vi "IHS.vi"() -> ()   [LabVIEW 2024]
doc: "This Labview program is made to run and administere the insect sampling system, using a Universal Robots UR-5 cobot. An Arduino Nano and the developd SRS system."
uses:
  SRS/controls/IHS_JKI.ctl
  <vilib>/userDefined/High Color/IMAQdx.ctl
  <vilib>/vision/Image Controls.llb/IMAQ Image.ctl
  <vilib>/addons/_JKI Toolkits/State Machine/_JKI_lib_State_Machine.llb/Select State(s)_err__jki_lib_state_machine.vi
  <vilib>/addons/_JKI Toolkits/State Machine/_JKI_lib_State_Machine.llb/Select State(s)_bool__jki_lib_state_machine.vi
  c074a71b-bfa2-4d9f-837e-66d7d0769231.vi
  <vilib>/addons/_JKI Toolkits/State Machine/_JKI_lib_State_Machine.llb/Periodic Trigger__ogtk__JKI-SM__jki_lib_state_machine.vi
  <vilib>/Utility/xml.llb/Write to XML File(string).vi
  <vilib>/vision/driver/NI_Vision_Acquisition_Software.lvlib
  <vilib>/vision/NI_Vision_Development_Module.lvlib
panel:
  in  "Force picture":bool
  in  "Force botton":bool
  in  "Simulate robot connection":bool
  in  "Training Picture":bool
  out "Num Before Next Pic":i32
  out "Executing Assignment":string
  out "Sample Num":i32
  in  "Save Settings":bool
  in  "Settings Button":bool
  out "Remote port":u16=30002
  out "UR-IP-address":string="192.168.0.10"
  out "Length":dbl
  out "CoM Y":dbl
  out "CoM X":dbl
  out "Orientation":dbl
  out "UR-Ready":bool
  out "Cam Connection":bool
  out "UR Connection":bool
  in  "Sample ID":string="Default"
  out "Robotmessage":string
  out "Number of objects":i32
  in  "Save Pictures":bool
  out "Vision A. Image":T1(plugin-control)
  out "Camera feed":T1(plugin-control)
  in  "Save Status His":bool
  out "Status History":string
  out "Insect-data-array":string[][](array[string])
  out "Status":string
  in  "Exit":bool
  in  "Pause Program":bool
  in  "Start Robot":bool
  # "Settings"
  # "Specimen info"
  # "-100°<RZ<100°"
  # "1.0mm<L<25.0mm"
  # "-0.750m<Y<0.750m"
  # "-0.750m<X<0.750m"
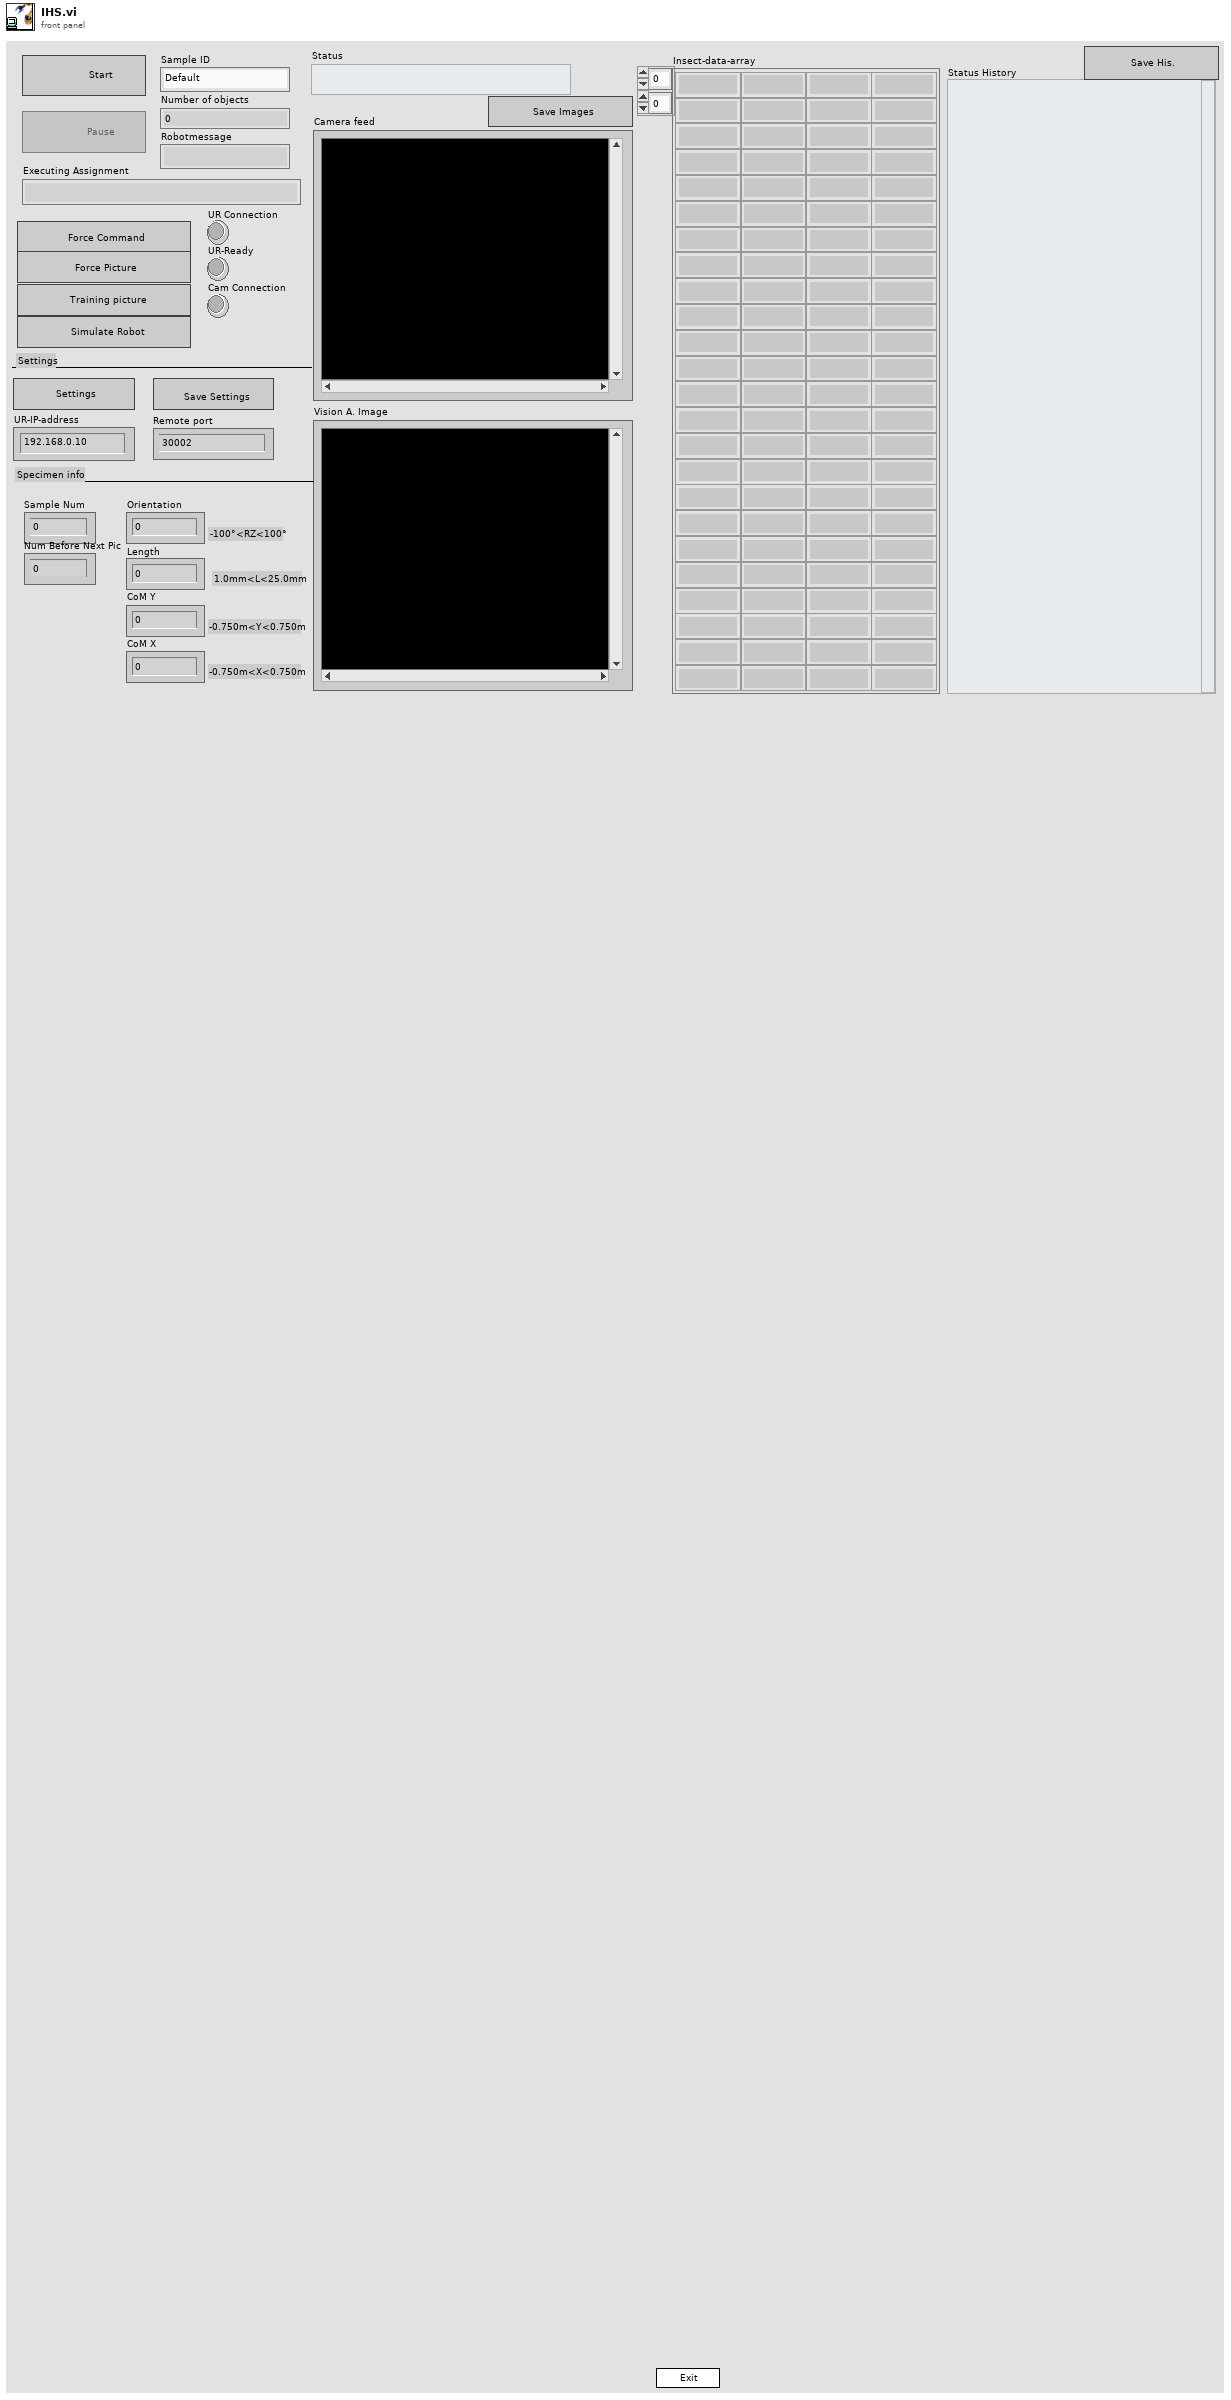
[diagram p1: front panel]
types:
  T1 = typedef "IMAQ Image.ctl" = refnum<image>
  T2 = typedef "IHS_JKI.ctl" = cluster{"Core":cluster{"Current VI Reference":refnum<vi>, "Close Panel on Exit?":bool, "Start Timestmap":string, "Status His":string, "Active":bool, "Exit":bool, "Assignment structure":string}, "Sample ID":string, "Cam":cluster{"Cam":T3, "Connected":bool, "Sim Image":bool, "Save pictures":bool}, "UR":cluster{"PC_IP":string, "Remote port":u16, "UR_IP":string, "connection ID":refnum<k5>, "Connected":bool, "Sim UR signal":bool, "UR Ready":bool, "Ready fail":dbl}, "Sample data":cluster{"Insects taken from current picture":i32, "Number of insects in pick-up area":i32, "Object data":cluster{"Object CoM X":dbl, "Object CoM Y":dbl, "Corrected Object orientation":dbl, "Object length":dbl, "Z, Height":dbl}, "Raw Particle Measurements":dbl[][], "Insect-data-array":string[][], "Sorted Particle Measurements":dbl[][], "Insects to pick this round":i32, "Picking array":dbl[][], "Pixels Measurements":dbl[][], "Tool1 to pick":i32}, "Images":cluster{"Image":T1, "Image Timestamp":string, "Boarder Image":T1, "Vision A. Image":T1}, "Reshake":i32, "Settings":cluster{"Number to try and pick":i32, "Last few":i32, "Z_Zero":dbl, "Tool switch size":dbl, "X-Zero":dbl, "Y-Zero":dbl, "Small or XL":dbl, "Tool1-Height":dbl, "Tool2-Height":dbl, "Ignore small":dbl, "Time to Whait":dbl}, "Assignment":cluster{"Executing Assignment":string, "Task":string, "Tool":string, "Specimen to pick":i32, "GO":bool}, "Return reason":string}
  T3 = typedef "IMAQdx.ctl" = refnum<k21>
  T4 = enum32{"Invalid", "Standard", "Closed", "Hidden", "Minimized", "Maximized"}
  T5 = enum32{"invalid app kind", "Development System", "Run Time System", "Student Edition", "Embedded LabVIEW", "Evaluation", "Custom"}
  T6 = enum8{"Enabled", "Disabled", "Disabled and Grayed Out"}
  T7 = enum16{"open", "replace", "create", "open or create", "replace or create", "replace or create with confirmation"}
  T8 = cluster{"Measurement Parameter":i32, "Range Lower Value":dbl, "Range Upper Value":dbl, "Range":bool, "Measurement Type":bool}
  T9 = cluster{"Left":i32, "Top":i32, "Right":i32, "Bottom":i32}
  T10 = cluster{"Measurement Parameter":i32, "Range Lower Value":dbl, "Range Upper Value":dbl, "Range":bool, "Measurement Type":bool}[]
  T11 = typedef "Image Type" = u32
  T12 = cluster{"Type":u32, "Version":u32, "Flags":u32, "SerialNumberHigh":u32, "SerialNumberLow":u32, "BusType":u32, "InterfaceName":string, "VendorName":string, "ModelName":string, "CameraFileName":string, "CameraAttributeURL":string}[]
  T13 = cluster{"Type":u32, "Version":u32, "Flags":u32, "SerialNumberHigh":u32, "SerialNumberLow":u32, "BusType":u32, "InterfaceName":string, "VendorName":string, "ModelName":string, "CameraFileName":string, "CameraAttributeURL":string}
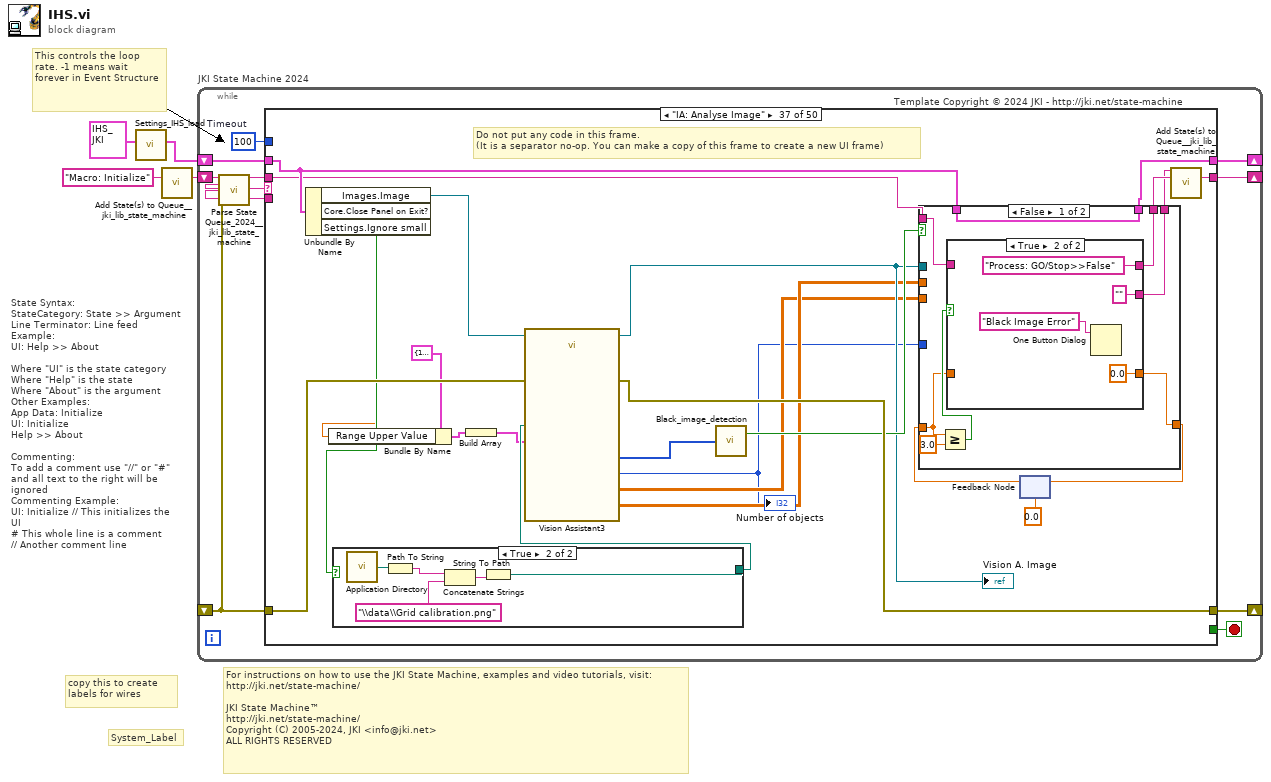
[diagram p0: block diagram]
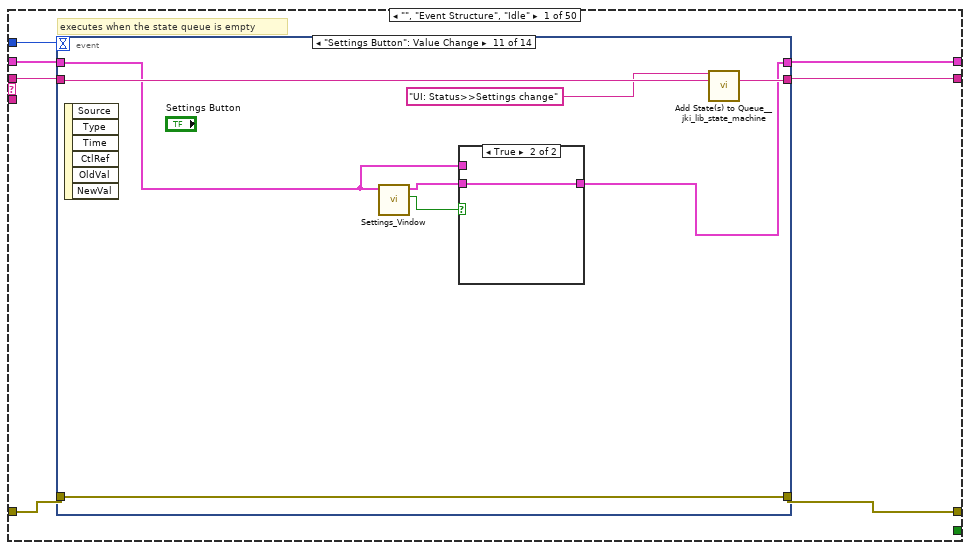
[diagram p2: hidden frame]
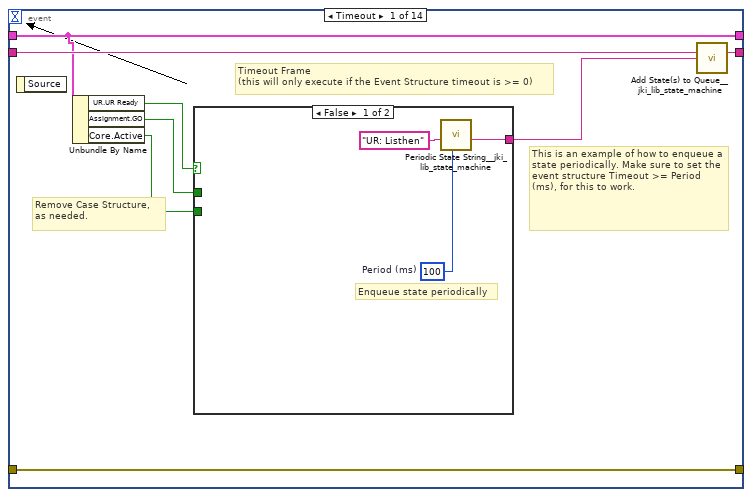
[diagram p3: hidden frame]
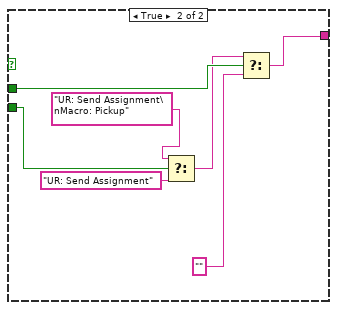
[diagram p4: hidden frame]
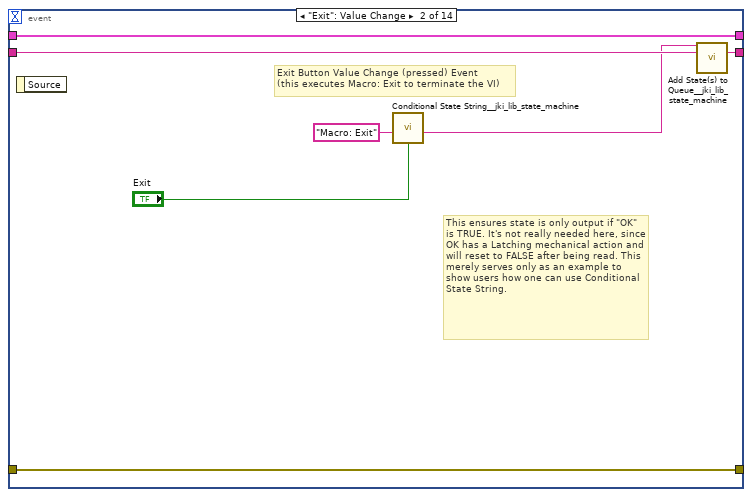
[diagram p5: hidden frame]
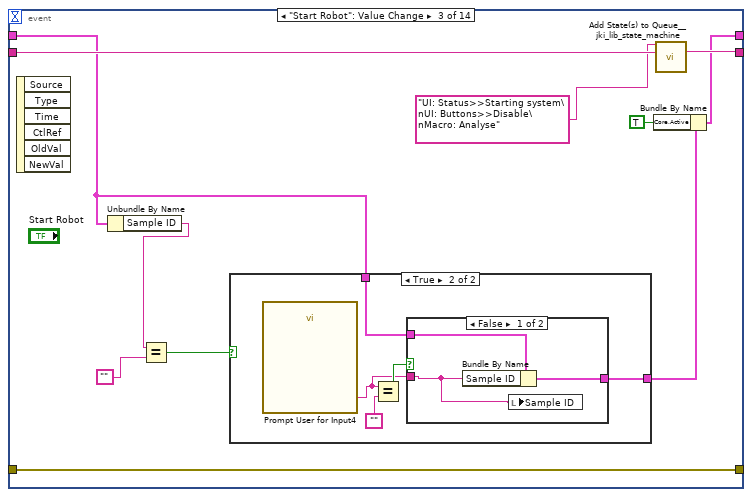
[diagram p6: hidden frame]
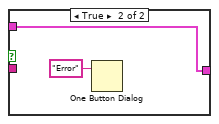
[diagram p8: hidden frame]
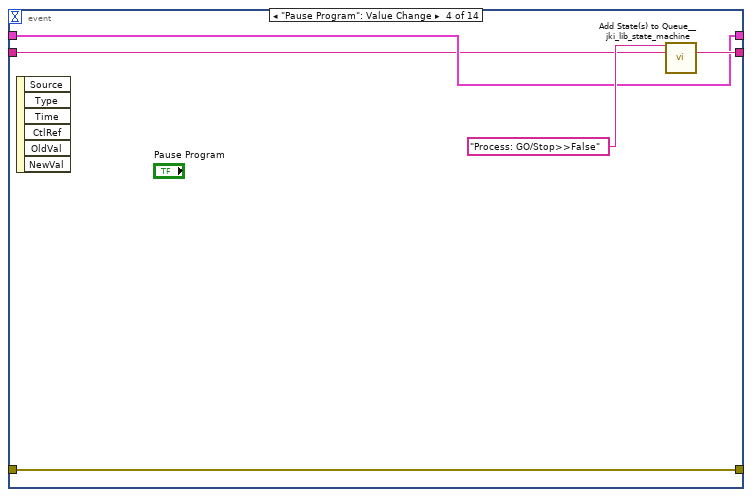
[diagram p9: hidden frame]
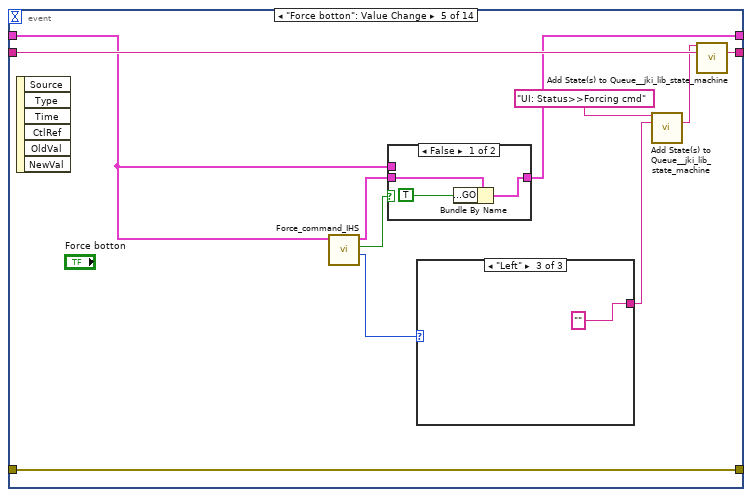
[diagram p10: hidden frame]
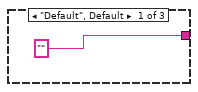
[diagram p11: hidden frame]
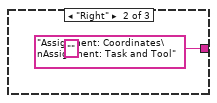
[diagram p12: hidden frame]
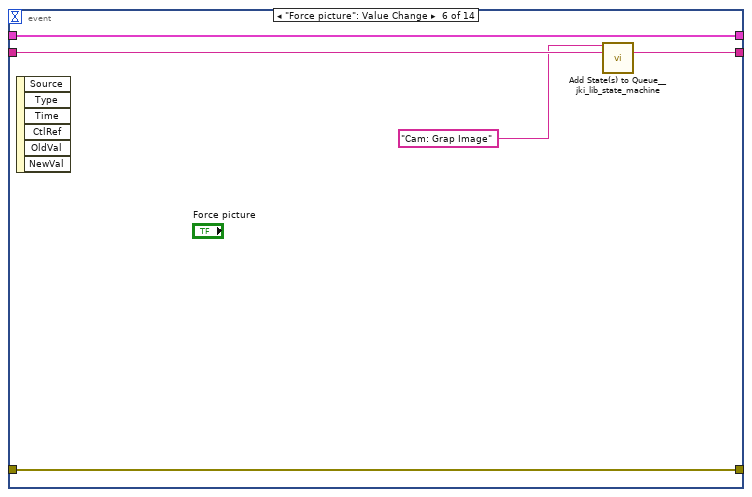
[diagram p14: hidden frame]
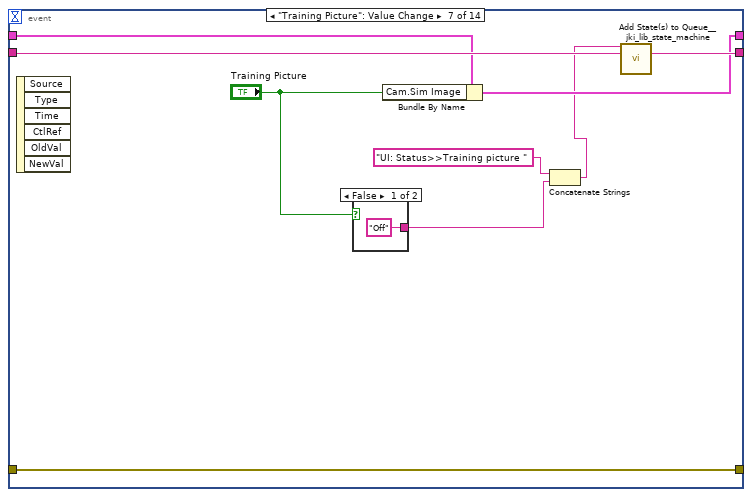
[diagram p15: hidden frame]
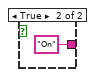
[diagram p16: hidden frame]
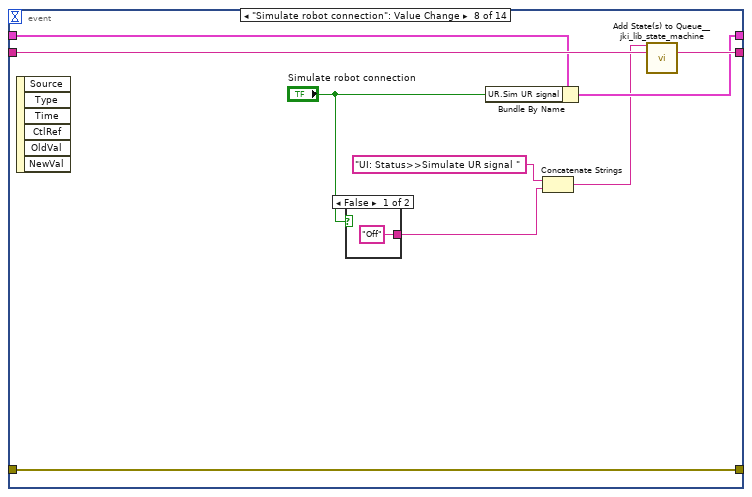
[diagram p17: hidden frame]
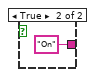
[diagram p18: hidden frame]
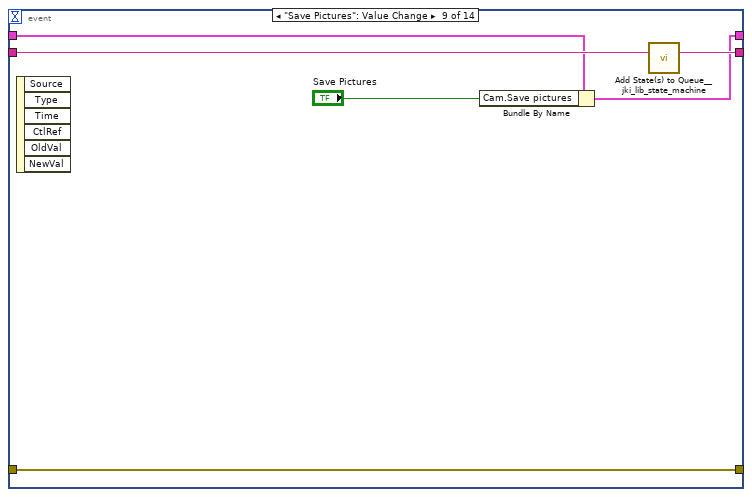
[diagram p19: hidden frame]
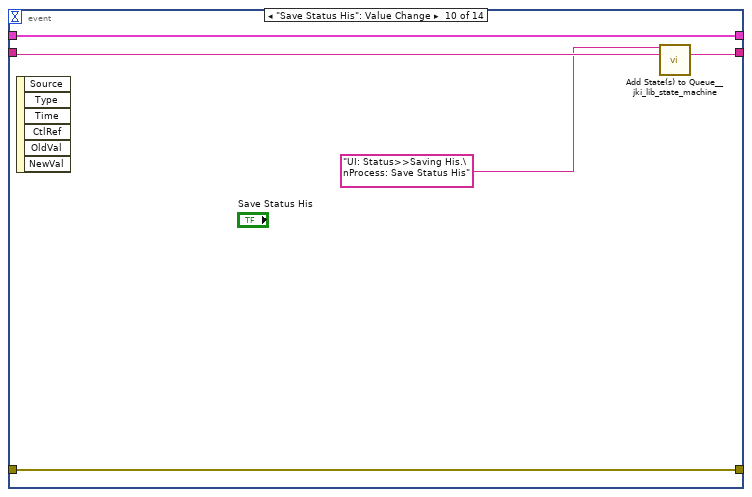
[diagram p20: hidden frame]
diagram:
  # "For instructions on how to use the JKI State Machine, examples and video tutorials, visit:\nhttp://jki.net/state-machine/\n\nJKI State Machine™\nhttp://jki.net/state-machine/\nCopyright (C) 2005-2024, JKI <info@jki.net>\nALL RIGHTS RESERVED"
  # "State Syntax:\nStateCategory: State >> Argument\nLine Terminator: Line feed\nExample:\nUI: Help >> About\n\nWhere \"UI\" is the state category\nWhere \"Help\" is the state\nWhere \"About\" is the argument\nOther Examples:\nApp Data: Initialize\nUI: Initialize\nHelp >> About\n\nCommenting:\nTo add a comment use \"//\" or \"#\" and all text to the right will be ignored\nCommenting Example:\nUI: Initialize // This initializes the UI\n# This whole line is a comment\n// Another comment line"
  # "copy this to create labels for wires"
  # "This controls the loop rate. -1 means wait forever in Event Structure"
  # "System_Label"
  n1 = call "Settings_IHS_load.vi"("Data IN"=T2 {"Core"={"Current VI Reference"=refnum, "Close Panel on Exit?"=FALSE, "Start Timestmap"="", "Status His"="", "Active"=FALSE, "Exit"=FALSE, "Assignment structure"="(Ta,To,X,Y,Z,0,0,O)"}, "Sample ID"="", "Cam"={"Cam"="", "Connected"=FALSE, "Sim Image"=FALSE, "Save pictures"=FALSE}, "UR"={"PC_IP"="192.168.0.15", "Remote port"=30002, "UR_IP"="192.168.0.10", "connection ID"=refnum, "Connected"=FALSE, "Sim UR signal"=FALSE, "UR Ready"=FALSE, "Ready fail"=0.0}, "Sample data"={"Insects taken from current picture"=0, "Number of insects in pick-up area"=0, "Object data"={"Object CoM X"=0.0, "Object CoM Y"=0.0, "Corrected Object orientation"=0.0, "Object length"=0.0, "Z, Height"=0.0}, "Raw Particle Measurements"=[], "Insect-data-array"=[], "Sorted Particle Measurements"=[], "Insects to pick this round"=0, "Picking array"=[], "Pixels Measurements"=[], "Tool1 to pick"=0}, "Images"={"Image"=refnum, "Image Timestamp"="", "Boarder Image"=refnum, "Vision A. Image"=refnum}, "Reshake"=0, "Settings"={"Number to try and pick"=8, "Last few"=4, "Z_Zero"=-104.5, "Tool switch size"=2.7, "X-Zero"=-39.3, "Y-Zero"=-392.7, "Small or XL"=12.0, "Tool1-Height"=-9.0, "Tool2-Height"=-12.5, "Ignore small"=0.5, "Time to Whait"=25.0}, "Assignment"={"Executing Assignment"="(0,0,0,0,0,0,0,0)", "Task"="0", "Tool"="0", "Specimen to pick"=0, "GO"=FALSE}, "Return reason"=""} ("Data")) -> ("Data OUT"=w2:T2)  [unwired: 9 in, 1 out]
  n2 = call <vilib>:"Add State(s) to Queue__jki_lib_state_machine.vi"("State(s) in (\"\")"="Macro: Initialize") -> ("States Out"=w4:string)  [unwired: 14 in]
  n3 = while "JKI State Machine 2024" {
    shift-right: [w9] -> _
    shift-left: w2 -> [w8]
    shift-right: [w11] -> _
    shift-left: _ -> [w6]
    shift-right: [w5] -> _
    shift-left: w4 -> [w12]
    stop <- w10 stop-if-true
    w7 = 100  # Timeout
    # "Template Copyright © 2024 JKI - http://jki.net/state-machine"
    n4 = call <vilib>:"Parse State Queue_2024__jki_lib_state_machine.vi"("State Queue"=w12, "Error In (no error)"=w6) -> ("Remaining States"=w14:string, "Current State"=w15:string, "Arguments"=w13:string)  [unwired: 11 in]
    n5 = case shown="\"IA: Analyse Image\"" w15 {
      selector: w15 -> [_ _ w161 _ _ _ _ _ _ _ _ _ _ _ _ _ _ _ _ _ _ _ _ _ _ _ _ _ _ _ _ _ _ _ _ _ _ _ _ _ _ _ _ _ _ _ _ _ _ _]
      tunnel: w14 -> [w22 w160 w165 w189 w199 w208 w212 w219 w230 w236 w240 w255 w274 w278 w284 w293 w304 w373 w378 w384 w398 w417 w421 w429 w438 w469 w481 w498 w516 w537 w541 w565 w589 w608 w641 w671 w683 w738 w778 w794 w830 w874 w903 w918 w936 w950 w968 w1019 w1061 w1075]
      tunnel: w13 -> [_ _ _ _ w194 _ _ _ _ _ _ _ w262 _ w279 w289 w298 _ _ _ _ _ _ w424 _ _ _ _ w511 _ _ _ _ _ _ _ _ _ _ _ _ _ _ _ _ _ _ _ _ _]
      tunnel: w8 -> [w20 w157 w163 w182 w196 w206 w209 w216 w222 w231 w237 w246 w261 w276 w282 w290 w300 w370 w375 w382 w392 w408 w418 w426 w436 w466 w477 w488 w514 w522 w538 w546 w584 w604 w622 w668 w689 w733 w775 w790 w825 w853 w882 w911 w933 w942 w963 w1011 w1056 w1070]
      tunnel: [w19 w158 w167 w186 errorcluster {"status"=FALSE, "code"=0, "source"=""} ("error out") w205 w210 w217 w220 w232 w238 w253 w272 w275 w280 w291 w301 w371 w376 w385 w396 w413 w419 w427 w443 w467 w479 w496 w512 w520 w539 w563 w587 w606 w639 w669 w692 w734 w776 w785 w827 w854 w877 w913 w934 w940 w965 w1016 w1059 w1071] -> w11
      tunnel: w6 -> [w16 w158 w166 w186 w195 w205 w210 w217 w221 w233 w238 w253 w272 w275 w281 w291 w302 w371 w376 w385 w396 w413 w419 w427 w443 w467 w479 w496 w513 w521 w539 w563 w587 w606 w639 w669 w693 w735 w776 w787 w828 w855 w880 w912 w934 w947 w966 w1017 w1059 w1072]
      tunnel: [w21 w159 w164 w188 w198 w207 w211 w218 w229 w235 w239 w254 w273 w277 w283 w292 w303 w372 w377 w386 w397 w416 w420 w428 w444 w468 w480 w497 w515 w536 w540 w564 w588 w607 w640 w670 w695 w737 w777 w793 w829 w873 w902 w917 w935 w949 w967 w1018 w1060 w1074] -> w5
      tunnel: [_ _ _ _ _ TRUE _ _ _ _ _ _ _ _ _ _ _ _ _ _ _ _ _ _ _ _ _ _ _ _ _ _ _ _ _ _ _ _ _ _ _ _ _ _ _ _ _ _ _ _] -> w10
      tunnel: [w18 w157 w163 w187 w196 w206 w209 w215 w222 w231 w237 w245 w260 w276 w282 w290 w300 w370 w375 w382 w394 w407 w418 w425 w442 w465 w476 w487 w514 w522 w538 w562 w585 w603 w638 w668 w684 w732 w775 w789 w826 w852 w882 w910 w933 w939 w962 w1010 w1058 w1073] -> w9
      tunnel: w7 -> [w17 _ _ _ _ _ _ _ _ _ _ _ _ _ _ _ _ _ _ _ _ _ _ _ _ _ _ _ _ _ _ _ _ _ _ _ _ _ _ _ _ _ _ _ _ _ _ _ _ _]
      frame "", "Event Structure", "Idle" {
        # "executes when the state queue is empty"
        n6 = event shown="[10] \"Settings Button\": Value Change" {
          selector: _ -> [_ _ _ _ _ _ _ _ _ _ _ _ _ _]
          dyn-events: _ -> [_ _ _ _ _ _ _ _ _ _ _ _ _ _]
          timeout: w17 -> [_ _ _ _ _ _ _ _ _ _ _ _ _ _]
          tunnel: w22 -> [w30 w47 w58 w70 w84 w96 w104 w116 w124 w129 w137 w142 w150 w156]
          tunnel: [w29 w46 w57 w74 w85 w95 w105 w117 w125 w130 w138 w143 w150 w155] -> w21
          tunnel: w20 -> [w27 w44 w54 w71 w82 w97 w103 w114 w122 w128 w132 w145 w148 w153]
          tunnel: [w28 w45 w56 w73 w78 w94 w106 w115 w123 w127 w133 w144 w149 w154] -> w19
          tunnel: w16 -> [w28 w45 w56 w73 w78 w94 w106 w115 w123 w127 w133 w144 w149 w154]
          tunnel: [w27 w44 w49 w71 w80 w97 w102 w113 w121 w128 w134 w145 w147 w153] -> w18
          event Timeout {
            # "Remove Case Structure, as needed."
            # "This is an example of how to enqueue a state periodically. Make sure to set the event structure Timeout >= Period (ms), for this to work."
            # "Timeout Frame\n(this will only execute if the Event Structure timeout is >= 0)"
            n7 = event-data() -> ()  [unwired: 1 in, 1 out]
            n8 = Unbundle By Name(w27) -> ("UR.UR Ready"=w26:bool, "Assignment.GO"=w25:bool, "Core.Active"=w23:bool)
            n9 = case shown="False" w26 {
              tunnel: [w33 w40] -> w24
              tunnel: w25 -> [_ w38]
              tunnel: w23 -> [_ w34]
              frame False {
                w32 = u32 100  # Period (ms)
                # "Enqueue state periodically"
                n10 = call <vilib>:"Periodic State String__jki_lib_state_machine.vi"("Period (ms)"=w32, "State"="UR: Listhen") -> ("State Out"=w33:string)  [unwired: 9 in]
              }
              frame True {
                n11 = Select(t="UR: Send Assignment\nMacro: Pickup", s=w34, f="UR: Send Assignment") -> (s? t:f=w35:string)
                n12 = Select(t=w35, s=w38, f="") -> (s? t:f=w40:string)
              }
            }
            n13 = call <vilib>:"Add State(s) to Queue__jki_lib_state_machine.vi"("State(s) in (\"\")"=w30, "State(s) at Back (\"\")"=w24) -> ("States Out"=w29:string)  [unwired: 13 in]
          }
          event "Exit": Value Change {
            # "This ensures state is only output if \"OK\" is TRUE. It's not really needed here, since OK has a Latching mechanical action and will reset to FALSE after being read. This merely serves only as an example to show users how one can use Conditional State String."
            # "Exit Button Value Change (pressed) Event\n(this executes Macro: Exit to terminate the VI)"
            n14 = event-data() -> ()  [unwired: 1 in, 1 out]
            n15 = call <vilib>:"Conditional State String__jki_lib_state_machine.vi"("Do State(s)?"="Exit", "State"="Macro: Exit") -> ("State Out"=w41:string)  [unwired: 7 in]
            n16 = call <vilib>:"Add State(s) to Queue__jki_lib_state_machine.vi"("State(s) in Front (\"\")"=w41, "State(s) in (\"\")"=w47) -> ("States Out"=w46:string)  [unwired: 13 in]
          }
          event "Start Robot": Value Change {
            n17 = event-data() -> ()  [unwired: 1 in, 6 out]
            n18 = Unbundle By Name(w54) -> ("Sample ID"=w52:string)
            n19 = Equal?(x=w52, y="") -> (x = y?=w51:bool)
            n20 = case shown="True" w51 {
              tunnel: w54 -> [w59 w62]
              tunnel: [w59 w61] -> w50
              frame False {
              }
              frame True {
                n21 = call "Prompt User for Input4"() -> ("Sample ID"=w60:string)  [unwired: 17 in, 2 out]
                n22 = Equal?(x=w60, y="") -> (x = y?=w63:bool)
                n23 = case shown="False" w63 {
                  tunnel: w62 -> [w67 w68]
                  tunnel: [w66 w68] -> w61
                  tunnel: w60 -> [w65 _]
                  frame False {
                    n24 = Bundle By Name(cluster=w67, "Sample ID"=w65) -> (w66:T2)
                    n25 = local write "Sample ID"(w65) -> ()
                  }
                  frame True {
                    n26 = One Button Dialog(message="Error") -> ()  [unwired: 1 in, 1 out]
                  }
                }
              }
            }
            n27 = Bundle By Name(cluster=w50, "Core.Active"=TRUE) -> (w49:T2)
            n28 = call <vilib>:"Add State(s) to Queue__jki_lib_state_machine.vi"("State(s) in Front (\"\")"="UI: Status>>Starting system\nUI: Buttons>>Disable\nMacro: Analyse" ("State(s) in Front (\"\")"), "State(s) in (\"\")"=w58) -> ("States Out"=w57:string)  [unwired: 13 in]
          }
          event "Pause Program": Value Change {
            n29 = event-data() -> ()  [unwired: 1 in, 6 out]
            n30 = call <vilib>:"Add State(s) to Queue__jki_lib_state_machine.vi"("State(s) in Front (\"\")"="Process: GO/Stop>>False" ("State(s) in Front (\"\")"), "State(s) in (\"\")"=w70) -> ("States Out"=w74:string)  [unwired: 13 in]
          }
          event "Force botton": Value Change {
            n31 = event-data() -> ()  [unwired: 1 in, 6 out]
            n32 = call "Force_command_IHS.vi"("Data In"=w82) -> ("Command type"=w79:enum16{"Default", "Right", "Left"}, "Canceled"=w83:bool, "Data Out"=w81:T2)  [unwired: 8 in]
            n33 = case shown="False" w83 {
              tunnel: w82 -> [_ w92]
              tunnel: w81 -> [w91 _]
              tunnel: [w90 w92] -> w80
              frame False {
                n34 = Bundle By Name(cluster=w91, "Assignment.GO"=TRUE) -> (w90:T2)
              }
              frame True {
              }
            }
            n35 = case shown="\"Left\"" w79 {
              tunnel: ["" ("State(s) in Front (\"\")") "" ("State(s) in Front (\"\")") "" ("State(s) in Front (\"\")")] -> w77
              frame "Default", Default {
              }
              frame "Right" {
                (unwired) "Assignment: Coordinates\nAssignment: Task and Tool" ("State(s) in Front (\"\")")
              }
              frame "Left" {
              }
            }
            n36 = call <vilib>:"Add State(s) to Queue__jki_lib_state_machine.vi"("State(s) in Front (\"\")"="UI: Status>>Forcing cmd" ("State(s) in Front (\"\")"), "State(s) in (\"\")"=w77) -> ("States Out"=w76:string)  [unwired: 13 in]
            n37 = call <vilib>:"Add State(s) to Queue__jki_lib_state_machine.vi"("State(s) in Front (\"\")"=w76, "State(s) in (\"\")"=w84) -> ("States Out"=w85:string)  [unwired: 13 in]
          }
          event "Force picture": Value Change {
            n38 = event-data() -> ()  [unwired: 1 in, 6 out]
            n39 = call <vilib>:"Add State(s) to Queue__jki_lib_state_machine.vi"("State(s) in Front (\"\")"="Cam: Grap Image" ("State(s) in Front (\"\")"), "State(s) in (\"\")"=w96) -> ("States Out"=w95:string)  [unwired: 13 in]
          }
          event "Training Picture": Value Change {
            n40 = event-data() -> ()  [unwired: 1 in, 6 out]
            n41 = case shown="False" "Training Picture" {
              tunnel: ["Off" ("string") "On" ("string")] -> w98
              frame False {
              }
              frame True {
              }
            }
            n42 = Bundle By Name(cluster=w103, "Cam.Sim Image"="Training Picture") -> (w102:T2)
            n43 = Concatenate Strings("UI: Status>>Training picture " ("State(s) in Front (\"\")"), w98) -> (w99:string)
            n44 = call <vilib>:"Add State(s) to Queue__jki_lib_state_machine.vi"("State(s) in Front (\"\")"=w99, "State(s) in (\"\")"=w104) -> ("States Out"=w105:string)  [unwired: 13 in]
          }
          event "Simulate robot connection": Value Change {
            n45 = event-data() -> ()  [unwired: 1 in, 6 out]
            n46 = case shown="False" "Simulate robot connection" {
              tunnel: ["Off" ("string") "On" ("string")] -> w111
              frame False {
              }
              frame True {
              }
            }
            n47 = Bundle By Name(cluster=w114, "UR.Sim UR signal"="Simulate robot connection") -> (w113:T2)
            n48 = Concatenate Strings("UI: Status>>Simulate UR signal " ("State(s) in Front (\"\")"), w111) -> (w110:string)
            n49 = call <vilib>:"Add State(s) to Queue__jki_lib_state_machine.vi"("State(s) in Front (\"\")"=w110, "State(s) in (\"\")"=w116) -> ("States Out"=w117:string)  [unwired: 13 in]
          }
          event "Save Pictures": Value Change {
            n50 = event-data() -> ()  [unwired: 1 in, 6 out]
            n51 = Bundle By Name(cluster=w122, "Cam.Save pictures"="Save Pictures") -> (w121:T2)
            n52 = call <vilib>:"Add State(s) to Queue__jki_lib_state_machine.vi"("State(s) in (\"\")"=w124) -> ("States Out"=w125:string)  [unwired: 14 in]
          }
          event "Save Status His": Value Change {
            n53 = event-data() -> ()  [unwired: 1 in, 6 out]
            n54 = call <vilib>:"Add State(s) to Queue__jki_lib_state_machine.vi"("State(s) in Front (\"\")"="UI: Status>>Saving His.\nProcess: Save Status His" ("State(s) in Front (\"\")"), "State(s) in (\"\")"=w129) -> ("States Out"=w130:string)  [unwired: 13 in]
          }
          event "Settings Button": Value Change {
            n55 = event-data() -> ()  [unwired: 1 in, 6 out]
            n56 = call "Settings_Vindow.vi"("Data"=w132) -> ("OK"=w135:bool, "output cluster"=w136:T2)  [unwired: 9 in]
            n57 = case shown="True" w135 {
              tunnel: w136 -> [_ w140]
              tunnel: [w139 w140] -> w134
              tunnel: w132 -> [w139 _]
              frame False {
              }
              frame True {
              }
            }
            n58 = call <vilib>:"Add State(s) to Queue__jki_lib_state_machine.vi"("State(s) in Front (\"\")"="UI: Status>>Settings change" ("State(s) in Front (\"\")"), "State(s) in (\"\")"=w137) -> ("States Out"=w138:string)  [unwired: 13 in]
          }
          event "Save Settings": Value Change {
            n59 = event-data() -> ()  [unwired: 1 in, 6 out]
            n60 = call <vilib>:"Add State(s) to Queue__jki_lib_state_machine.vi"("State(s) in Front (\"\")"="UI: Status>>Saving settings\nData: Save Settings" ("State(s) in Front (\"\")"), "State(s) in (\"\")"=w142) -> ("States Out"=w143:string)  [unwired: 13 in]
          }
          event "Sample ID": Value Change {
            n61 = event-data() -> ()  [unwired: 1 in, 6 out]
            n62 = Bundle By Name(cluster=w148, "Sample ID"="Sample ID") -> (w147:T2)
          }
          event Panel Close? {
            # "Discard the event because we'll close the front panel ourselves in Macro: Exit"
            # "Close Panel button (pressed) Event\n(this executes Macro: Exit to terminate the VI)"
            n63 = event-data() -> ()  [unwired: 1 in, 1 out]
            n64 = event-data("Discard?"=TRUE) -> ()  [unwired: 1 in, 1 out]
            n65 = call <vilib>:"Add State(s) to Queue__jki_lib_state_machine.vi"("State(s) in Front (\"\")"="Macro: Exit", "State(s) in (\"\")"=w156) -> ("States Out"=w155:string)  [unwired: 13 in]
          }
        }
      }
      frame "---------- Core ----------" {
        # "Do not put any code in this frame.\n(it is a separator no-op)"
        n66 = call <vilib>:"Add State(s) to Queue__jki_lib_state_machine.vi"("State(s) in (\"\")"=w160) -> ("States Out"=w159:string)  [unwired: 14 in]
      }
      frame Default {
        w170 = 42 items=["No error", "Argument error", "Memory is full", "Out of zone", "End of file", "File already open", "Generic file I/O error", "File not found", "File permission error", "Disk is full", "Duplicate path", "Too many files open", "System feature not enabled", "Resource file not found", "Cannot add resource", "Resource not found", "Image not found", "Image memory error", "Pen does not exist", "Config type invalid", "Config token not found", "Config parse error", "Config memory error", "Bad external code format", "Bad external code offset", "External code not present", "Null window", "Destroy window error", "Null menu", "Print aborted", "Bad print record", "Print driver error", "Windows error during printing", "Memory error during printing", "Print dialog error", "Generic print error", "Invalid device refnum", "Device not found", "Device parameter error", "Device unit error", "Cannot open device", "Device call aborted", "Generic error", "Cancelled by user", "Object ID too low", "Object ID too high", "Object not in heap", "Unknown heap", "Unknown object (invalid DefProc)", "Unknown object (DefProc not in table)", "Message out of range", "Invalid (null) method", "Unknown message", "Manager call not supported", "Bad address", "Network operation in progress", "Network operation timed out", "Connection is busy", "Network attribute not supported", "Network error", "Address in use", "System out of memory", "Connection aborted", "Connection refused", "Not connected", "Already connected", "Connection closed", "Initialization error (interapplication manager)", "Bad occurrence", "Wait on unbound occurrence handler", "Occurrence queue overflow", "Datalog type conflict", "Unused", "Unrecognized type (interapplication manager)", "Memory corrupt", "Failed to make temporary DLL", "Old CIN version", "Drag socket not found", "Failed to load drop-object", "Failed to register OLE object", "Failed to release OLE object", "Format specifier type mismatch", "Unknown format specifier", "Too few format specifiers", "Too many format specifiers", "Scan failed", "Newer CIN version", "Error converting to variant", "Runtime menu error", "Password tampered", "Variant attribute not found", "Incompatible variant data type", "Event data is not available", "Event Store is not present", "Occurrence is not found", "Event Queue is not created", "Event info is not available", "Refnum passed is NULL", "Error retrieving Class GUID", "Error retrieving CoClass GUID", "Error retrieving TypeLib GUID.", "Bad built application magic bytes.", "Specific driver is different from the specific driver associated with the Logical Name.", "There is no session opened to the class driver.", "Max Error", "MAX - Error with config objects", "MAX - Error loading configuration", "MAX - Group not supported"]
        # "Current State"
        # "Do not delete, rename, or modify this frame.\n(this is used to capture unhandled states and typos)"
        # "Handle mistyped state name (developer tool)"
        n67 = Format Into String(format string="Software Exception: Unhandled State \"%s\"." ("message"), error in=w166, w161) -> (resulting string=w169:string, error out=w168:errorcluster)  [unwired: 1 in]
        n68 = call <vilib>:"Error Cluster From Error Code.vi"("show call chain? (False)"=TRUE, "error in (no error)"=w168, "error message (\"\")"=w169, "error code (0)"=w170) -> ("error out"=w167:errorcluster)  [unwired: 5 in]
        n69 = call <vilib>:"Add State(s) to Queue__jki_lib_state_machine.vi"("State(s) in (\"\")"=w165) -> ("States Out"=w164:string)  [unwired: 14 in]
      }
      frame "Initialize Core Data" {
        w172 = FALSE ("Save Pictures")
        w173 = FALSE ("Cam.Connected")
        # "Do not delete, rename, or modify this frame.\n(this is used to determine panel behavior on exit)"
        # "originally closed?"
        # "exe?"
        # "If panel starts closed or is an EXE, then close it when we exit"
        n70 = property class="VI"() -> ("FP.State"=w179:T4)  [unwired: 2 in, 2 out]
        n71 = property class="App"() -> ("App.Kind"=w185:T5)  [unwired: 2 in, 2 out]
        n72 = control-ref of="Current VI Reference"() -> (w180:refnum<vi>)
        n73 = Equal?(x=w179, y=T4."Closed" ("Front Panel Window:State")) -> (x = y?=w177:bool)
        n74 = Equal?(x=w185, y=T5."Run Time System" ("Application:Kind")) -> (x = y?=w183:bool)
        n75 = Or(x=w177, y=w183) -> (x .or. y?=w181:bool)
        n76 = property on="Simulate robot connection" class="Bool (strict)"("Value"=w172) -> ()  [unwired: 2 in, 2 out]
        n77 = property on="Training Picture" class="Bool (strict)"("Value"=w172) -> ()  [unwired: 2 in, 2 out]
        n78 = property on="Save Pictures" class="Bool (strict)"("Value"=w172) -> ()  [unwired: 2 in, 2 out]
        n79 = Format Date/Time String(time format string (%c)="%y%m%d-%H;%M;%S") -> (date/time string=w175:string)  [unwired: 2 in]
        n80 = Bundle By Name(cluster=w182, "Core.Current VI Reference"=w180, "Core.Close Panel on Exit?"=w181, "Core.Start Timestmap"=w175, "Core.Status His"="", "Cam.Connected"=w173, "Cam.Connected"=w173, "Cam.Save pictures"=w173, "UR.UR Ready"=w173, "UR.Sim UR signal"=w173, "Cam.Sim Image"=w173) -> (w187:T2)
        n81 = call <vilib>:"Add State(s) to Queue__jki_lib_state_machine.vi"("State(s) in (\"\")"=w189) -> ("States Out"=w188:string)  [unwired: 14 in]
      }
      frame "Error Handler" {
        # "When running as sourcecode, this function will add previous state data to the error message to aid the developer in troubleshoot errors.\nIf run as an executable, no additional information is added to the error message."
        # "This state receives both Errors and Warnings which is how the Status of this wire can be FALSE"
        # "Unhandled Error -- Display it"
        # "Handle any errors or warnings here.\nYou can also output any states to clean-up after errors or warnings occur"
        # "Clear error or warning"
        n82 = disable-structure shown="Default" {
          disable-tunnel: w195 -> [w202 w203]
          disable-tunnel: w194 -> [w201 _]
          disable-tunnel: [w200 w203] -> w193
          frame condition #0 (active) {
            n83 = call <vilib>:"Append Error Details__jki_lib_state_machine.vi"("error in (no error)"=w202, "Previous State and Argument(s)"=w201) -> ("error out"=w200:errorcluster)  [unwired: 9 in]
          }
          frame condition #1 {
          }
        }
        n84 = call <vilib>:"General Error Handler.vi"("error in (no error)"=w193) -> ()  [unwired: 10 in, 5 out]
        n85 = call-poly <vilib>:"Select State(s)__jki_lib_state_machine.vi"("State(s) if True (\"\")"="/* Post Error States", "Select"=w193, "State(s) if False (\"\")"="/* Post Warning States") -> ("States Out"=w191:string)  [unwired: 12 in]
        n86 = call <vilib>:"Add State(s) to Queue__jki_lib_state_machine.vi"("State(s) in Front (\"\")"=w191, "State(s) in (\"\")"=w199) -> ("States Out"=w198:string)  [unwired: 13 in]
      }
      frame "Exit" {
        # "Do not put any code in this frame.\n(No errors that occur here will be handled.)"
        n87 = call <vilib>:"Add State(s) to Queue__jki_lib_state_machine.vi"("State(s) in (\"\")"=w208) -> ("States Out"=w207:string)  [unwired: 14 in]
      }
      frame "---------- Data ----------" {
        # "Do not put any code in this frame.\n(It is a separator no-op. You can make a copy of this frame to create a new Data frame)"
        n88 = call <vilib>:"Add State(s) to Queue__jki_lib_state_machine.vi"("State(s) in (\"\")"=w212) -> ("States Out"=w211:string)  [unwired: 14 in]
      }
      frame "Data: Initialize" {
        w214 = TRUE  # Close Panel on Exit?
        w213 = refnum<vi> refnum  # Current VI Reference
        # "Initialize the shift-register data, here.\n(data names are defined by what you wire into the bundle function)"
        n89 = Bundle By Name(cluster=w216, "Core.Current VI Reference"=w213, "Core.Close Panel on Exit?"=w214) -> (w215:T2)
        n90 = call <vilib>:"Add State(s) to Queue__jki_lib_state_machine.vi"("State(s) in (\"\")"=w219) -> ("States Out"=w218:string)  [unwired: 14 in]
      }
      frame "Data: Save Settings" {
        # "Do not put any code in this frame.\n(It is a separator no-op. You can make a copy of this frame to create a new Data frame)"
        n91 = call <vilib>:"Application Directory.vi"() -> ("Application Directory"=w226:path)
        n92 = Path To String(path=w226) -> (string=w227:string)
        n93 = Concatenate Strings(w227, "\\settings-IHS.ini" ("string")) -> (w224:string)
        n94 = String To Path(string=w224) -> (path=w223:path)
        n95 = Flatten To XML(6:w222) -> (2:w228:string)
        n96 = call-poly <vilib>:"Write to XML File.vi"("error in (no error)"=w221, "XML Input"=w228, "XML File Path"=w223) -> ("error out"=w220:errorcluster)  [unwired: 6 in, 2 out]
        n97 = call <vilib>:"Add State(s) to Queue__jki_lib_state_machine.vi"("State(s) in (\"\")"=w230) -> ("States Out"=w229:string)  [unwired: 14 in]
      }
      frame "Data: Cleanup" {
        # "Cleanup any data and references, here.\n(this is called automatically, by the Macro: Exit)"
        n98 = Unbundle By Name(w231) -> ("Core.Current VI Reference"=w234:refnum<vi>)
        n99 = Close Reference(reference=w234, error in (no error)=w233) -> (error out=w232:errorcluster)
        n100 = call <vilib>:"Add State(s) to Queue__jki_lib_state_machine.vi"("State(s) in (\"\")"=w236) -> ("States Out"=w235:string)  [unwired: 14 in]
      }
      frame "---------- UI ----------" {
        # "Do not put any code in this frame.\n(It is a separator no-op. You can make a copy of this frame to create a new UI frame)"
        n101 = call <vilib>:"Add State(s) to Queue__jki_lib_state_machine.vi"("State(s) in (\"\")"=w240) -> ("States Out"=w239:string)  [unwired: 14 in]
      }
      frame "UI: Initialize" {
        w241 = FALSE ("UR Connection")
        w247 = "" ("Status History")
        w249 = 0.0 ("Object length 2")
        # "Initialize the User Interface, here.\n(this is called automatically, by the Macro: Initialize)"
        n102 = Unbundle By Name(w246) -> ("UR.UR_IP"=→"UR-IP-address":string, "UR.Remote port"=→"Remote port":u16)
        n103 = local write "Status History"(w247) -> ()
        n104 = local write "Status"(w247) -> ()
        n105 = local write "Insect-data-array"(string[][] []) -> ()
        n106 = local write "Number of objects"(0 ("Number of objects")) -> ()
        n107 = local write "Length"(w249) -> ()
        n108 = local write "CoM Y"(w249) -> ()
        n109 = local write "CoM X"(w249) -> ()
        n110 = local write "Orientation"(w249) -> ()
        n111 = local read "Sample ID"() -> (w242:string)
        n112 = Not Equal?(x=w242, y="Default") -> (x != y?=w244:bool)
        n113 = case shown="False" w244 {
          tunnel: w246 -> [w256 w259]
          tunnel: [w256 w258] -> w245
          tunnel: w242 -> [_ w257]
          frame False {
          }
          frame True {
            n114 = Bundle By Name(cluster=w259, "Sample ID"=w257) -> (w258:T2)
          }
        }
        n115 = property on="Cam Connection" class="Bool (strict)"("Value"=w241) -> ()  [unwired: 2 in, 2 out]
        n116 = property on="UR Connection" class="Bool (strict)"("Value"=w241) -> ()  [unwired: 2 in, 2 out]
        n117 = property on="UR-Ready" class="Bool (strict)"("Value"=w241) -> ()  [unwired: 2 in, 2 out]
        n118 = call <vilib>:"Add State(s) to Queue__jki_lib_state_machine.vi"("State(s) in (\"\")"=w255) -> ("States Out"=w254:string)  [unwired: 14 in]
      }
      frame "UI: Status" {
        # "Do not put any code in this frame.\n(It is a separator no-op. You can make a copy of this frame to create a new UI frame)"
        n119 = Unbundle By Name(w261) -> ("Core.Start Timestmap"=w263:string)
        n120 = Concatenate Strings("Starting system", w263) -> (w267:string)
        n121 = Format Date/Time String(time format string (%c)="%H;%M;%S") -> (date/time string=w264:string)  [unwired: 2 in]
        n122 = call <vilib>:"Space Constant.vi"() -> ("String"=w265:string)
        n123 = feedback #1(w267) -> (w270:string)
        n124 = Concatenate Strings(w270, "\r\n", w264, w265, w262) -> (w269:string)
        "Status History" <- w269
        n125 = feedback-in #1(w269) -> ()
        n126 = Bundle By Name(cluster=w261, "Core.Status His"=w269) -> (w260:T2)
        n127 = call <vilib>:"Add State(s) to Queue__jki_lib_state_machine.vi"("State(s) in (\"\")"=w274) -> ("States Out"=w273:string)  [unwired: 14 in]
        "Status" <- w262
      }
      frame "UI: Uninitialize" {
        # "Cleanup the User Interface, here.\n(this is called automatically, by the Macro: Exit)"
        n128 = call <vilib>:"Add State(s) to Queue__jki_lib_state_machine.vi"("State(s) in (\"\")"=w278) -> ("States Out"=w277:string)  [unwired: 14 in]
      }
      frame "UI: Cursor Set" {
        # "Argument"
        # "Set and Unset Cursor Busy.\n(Usage: \"UI: Cursor Set >> Busy|Idle\")"
        n129 = case shown="\"Idle\", Default" w279 {
          tunnel: w281 -> [w286 w288]
          tunnel: [w285 w287] -> w280
          frame "Idle", Default {
            n130 = call <vilib>:"Unset Busy.vi"("error in (no error)"=w286) -> ("error out"=w285:errorcluster)  [unwired: 10 in]
          }
          frame "Busy" {
            n131 = call <vilib>:"Set Busy.vi"("error in (no error)"=w288) -> ("error out"=w287:errorcluster)  [unwired: 9 in, 1 out]
          }
        }
        n132 = call <vilib>:"Add State(s) to Queue__jki_lib_state_machine.vi"("State(s) in (\"\")"=w284) -> ("States Out"=w283:string)  [unwired: 14 in]
      }
      frame "UI: Buttons" {
        # "Do not put any code in this frame.\n(It is a separator no-op. You can make a copy of this frame to create a new UI frame)"
        n133 = case shown="\"Enable\", Default" w289 {
          frame "Enable", Default {
            w294 = T6."Enabled" ("Disabled")
            n134 = property on="Start Robot" class="Bool"("DisabledEnum"=w294) -> ()  [unwired: 2 in, 2 out]
            n135 = property on="Force botton" class="Bool"("DisabledEnum"=w294) -> ()  [unwired: 2 in, 2 out]
            n136 = property on="Save Pictures" class="Bool (strict)"("DisabledEnum"=w294) -> ()  [unwired: 2 in, 2 out]
            n137 = property on="Training Picture" class="Bool (strict)"("DisabledEnum"=w294) -> ()  [unwired: 2 in, 2 out]
            n138 = property on="Save Status His" class="Bool"("DisabledEnum"=w294) -> ()  [unwired: 2 in, 2 out]
            n139 = property on="Settings Button" class="Bool"("DisabledEnum"=w294) -> ()  [unwired: 2 in, 2 out]
            n140 = property on="Save Settings" class="Bool"("DisabledEnum"=w294) -> ()  [unwired: 2 in, 2 out]
            n141 = property on="Simulate robot connection" class="Bool (strict)"("DisabledEnum"=w294) -> ()  [unwired: 2 in, 2 out]
            n142 = property on="Pause Program" class="Bool"("DisabledEnum"=T6."Disabled and Grayed Out" ("Disabled")) -> ()  [unwired: 2 in, 2 out]
          }
          frame "Disable" {
            w296 = T6."Disabled and Grayed Out" ("Disabled")
            n143 = property on="Start Robot" class="Bool"("DisabledEnum"=w296) -> ()  [unwired: 2 in, 2 out]
            n144 = property on="Force botton" class="Bool"("DisabledEnum"=w296) -> ()  [unwired: 2 in, 2 out]
            n145 = property on="Save Pictures" class="Bool (strict)"("DisabledEnum"=w296) -> ()  [unwired: 2 in, 2 out]
            n146 = property on="Training Picture" class="Bool (strict)"("DisabledEnum"=w296) -> ()  [unwired: 2 in, 2 out]
            n147 = property on="Save Status His" class="Bool"("DisabledEnum"=w296) -> ()  [unwired: 2 in, 2 out]
            n148 = property on="Settings Button" class="Bool"("DisabledEnum"=w296) -> ()  [unwired: 2 in, 2 out]
            n149 = property on="Save Settings" class="Bool"("DisabledEnum"=w296) -> ()  [unwired: 2 in, 2 out]
            n150 = property on="Simulate robot connection" class="Bool (strict)"("DisabledEnum"=w296) -> ()  [unwired: 2 in, 2 out]
            n151 = property on="Pause Program" class="Bool"("DisabledEnum"=T6."Enabled" ("Disabled")) -> ()  [unwired: 2 in, 2 out]
          }
        }
        n152 = call <vilib>:"Add State(s) to Queue__jki_lib_state_machine.vi"("State(s) in (\"\")"=w293) -> ("States Out"=w292:string)  [unwired: 14 in]
      }
      frame "UI: Front Panel State" {
        # "Argument"
        # "Set Front Panel Open or Closed\n(Usage: \"UI: Front Panel State >> Open|Close\")"
        n153 = Unbundle By Name(w300) -> ("Core.Current VI Reference"=w299:refnum<vi>)
        n154 = case shown="\"Maximize\", \"Maximized\"" w298 {
          tunnel: w302 -> [w310 w325 w336 w349 w362]
          tunnel: [w312 w326 w338 w351 w364] -> w301
          tunnel: w299 -> [w311 w323 w337 w350 w363]
          frame "Open", "Standard", Default {
            w305 = T4."Standard" ("State")
            n155 = property class="VI"(reference=w311, error in=w310) -> (reference out=w308:refnum<vi>, error out=w309:errorcluster, "FP.State"=w307:T4)
            n156 = Not Equal?(x=w307, y=w305) -> (x != y?=w306:bool)
            n157 = case shown="True" w306 {
              tunnel: [w316 w318] -> w312
              tunnel: w309 -> [w315 w318]
              tunnel: w308 -> [w314 _]
              tunnel: w305 -> [w313 _]
              frame True {
                n158 = invoke class="VI" method="FP.Open"(reference=w314, error in=w315, "Activate"=TRUE, "State"=w313) -> (error out=w316:errorcluster)  [unwired: 1 in, 4 out]
              }
              frame False {
              }
            }
          }
          frame "Close", "Closed" {
            n159 = property class="VI"(reference=w323, error in=w325) -> (reference out=w322:refnum<vi>, error out=w324:errorcluster, "FP.State"=w320:T4)
            n160 = Not Equal?(x=w320, y=T4."Closed" ("Front Panel Window:State")) -> (x != y?=w319:bool)
            n161 = case shown="True" w319 {
              tunnel: [w327 w330] -> w326
              tunnel: w324 -> [w327 w329]
              tunnel: w322 -> [_ w328]
              frame False {
              }
              frame True {
                n162 = invoke class="VI" method="FP.Close"(reference=w328, error in=w329) -> (error out=w330:errorcluster)  [unwired: 1 in, 2 out]
              }
            }
          }
          frame "Hidden", "Hide" {
            w331 = T4."Hidden" ("State")
            n163 = property class="VI"(reference=w337, error in=w336) -> (reference out=w334:refnum<vi>, error out=w335:errorcluster, "FP.State"=w333:T4)
            n164 = Not Equal?(x=w333, y=w331) -> (x != y?=w332:bool)
            n165 = case shown="True" w332 {
              tunnel: [w342 w343] -> w338
              tunnel: w335 -> [w341 w343]
              tunnel: w334 -> [w340 _]
              tunnel: w331 -> [w339 _]
              frame True {
                n166 = invoke class="VI" method="FP.Open"(reference=w340, error in=w341, "State"=w339) -> (error out=w342:errorcluster)  [unwired: 2 in, 4 out]
              }
              frame False {
              }
            }
          }
          frame "Minimize", "Minimized" {
            w344 = T4."Minimized" ("State")
            n167 = property class="VI"(reference=w350, error in=w349) -> (reference out=w347:refnum<vi>, error out=w348:errorcluster, "FP.State"=w346:T4)
            n168 = Not Equal?(x=w346, y=w344) -> (x != y?=w345:bool)
            n169 = case shown="True" w345 {
              tunnel: [w355 w356] -> w351
              tunnel: w348 -> [w354 w356]
              tunnel: w347 -> [w353 _]
              tunnel: w344 -> [w352 _]
              frame True {
                n170 = invoke class="VI" method="FP.Open"(reference=w353, error in=w354, "State"=w352) -> (error out=w355:errorcluster)  [unwired: 2 in, 4 out]
              }
              frame False {
              }
            }
          }
          frame "Maximize", "Maximized" {
            w357 = T4."Maximized" ("State")
            n171 = property class="VI"(reference=w363, error in=w362) -> (reference out=w360:refnum<vi>, error out=w361:errorcluster, "FP.State"=w359:T4)
            n172 = Not Equal?(x=w359, y=w357) -> (x != y?=w358:bool)
            n173 = case shown="False" w358 {
              tunnel: [w368 w369] -> w364
              tunnel: w361 -> [w367 w369]
              tunnel: w360 -> [w366 _]
              tunnel: w357 -> [w365 _]
              frame True {
                n174 = invoke class="VI" method="FP.Open"(reference=w366, error in=w367, "State"=w365) -> (error out=w368:errorcluster)  [unwired: 2 in, 4 out]
              }
              frame False {
              }
            }
          }
        }
        n175 = call <vilib>:"Add State(s) to Queue__jki_lib_state_machine.vi"("State(s) in (\"\")"=w304) -> ("States Out"=w303:string)  [unwired: 14 in]
      }
      frame "---------- Macro ----------" {
        # "Do not put any code in this frame.\n(It is a separator no-op. You can make a copy of this frame to create a new Macro frame)"
        n176 = call <vilib>:"Add State(s) to Queue__jki_lib_state_machine.vi"("State(s) in (\"\")"=w373) -> ("States Out"=w372:string)  [unwired: 14 in]
      }
      frame "Macro: Initialize" {
        w374 = "UI: Cursor Set>>Busy\nData: Initialize\nInitialize Core Data\nUI: Initialize\nUI: Buttons>>Enable\nUI: Front Panel State >>Maximize\nUR: Initialize\nUR: Listhen\nCam: Initialize\nUI: Status>>Wellcome\nUI: Cursor Set>>Idle"  # UI: Cursor Set>>Busy Data: Initialize Initialize Core Data UI: Initialize UI: Buttons>>Enable UI: Front Panel State >>Maximize UR: Initialize UR: Listhen Cam: Initialize UI: Status>>Wellcome UI: Cursor Set>>Idle
        # "Initialization Macro\n(This is called once, when the VI starts)"
        n177 = call <vilib>:"Add State(s) to Queue__jki_lib_state_machine.vi"("State(s) in Front (\"\")"=w374, "State(s) in (\"\")"=w378) -> ("States Out"=w377:string)  [unwired: 13 in]
      }
      frame "Macro: Analyse" {
        # "Do not put any code in this frame.\n(It is a separator no-op. You can make a copy of this frame to create a new Macro frame)"
        n178 = Unbundle By Name(w382) -> ("Cam.Sim Image"=w381:bool)
        n179 = call-poly <vilib>:"Select State(s)__jki_lib_state_machine.vi"("State(s) if True (\"\")"="UI: Cursor Set>>Busy\nAssignment: Distangle\nCam: Select test image\nIA: Analyse Image\nProcess: Check for Objects\nProcess: Reshape Array\nProcess: Clear Sample Data\nProcess: Choose tool\nIA: Draw borders\nUI: Cursor Set>>Idle\nMacro: Pickup" ("State(s) in Front (\"\")"), "Select"=w381, "State(s) if False (\"\")"="UI: Cursor Set>>Busy\nAssignment: Distangle\nAssignment: Cam Pos\nCam: Grap Image\nIA: Analyse Image\nProcess: Check for Objects\nProcess: Reshape Array\nProcess: Clear Sample Data\nProcess: Choose tool\nIA: Draw borders\nUI: Cursor Set>>Idle\nMacro: Pickup" ("State(s) in Front (\"\")")) -> ("States Out"=w383:string)  [unwired: 12 in]
        n180 = call <vilib>:"Add State(s) to Queue__jki_lib_state_machine.vi"("State(s) in Front (\"\")"=w383, "State(s) in (\"\")"=w384) -> ("States Out"=w386:string)  [unwired: 13 in]
      }
      frame "Macro: Pickup" {
        # "Do not put any code in this frame.\n(It is a separator no-op. You can make a copy of this frame to create a new Macro frame)"
        n181 = Unbundle By Name(w392) -> ("Sample data.Insects to pick this round"=w387:i32, "Sample data.Insects taken from current picture"=w389:i32, "Cam.Sim Image"=w391:bool)
        "Sample Num" <- w389
        n182 = Subtract(x=w387, y=w389) -> (x-y=→"Num Before Next Pic":i32)
        n183 = Greater Or Equal?(x=w389, y=w387) -> (x >= y?=w390:bool)
        n184 = case shown="False" w390 {
          tunnel: ["Assignment: Coordinates\nAssignment: Task and Tool" ("State(s) in Front (\"\")") w403] -> w395
          tunnel: w391 -> [_ w401]
          tunnel: [TRUE FALSE] -> w388
          frame False {
            # "To allow for the system to run better\nThese commands are first put in que,\nwhen the system detects done from UR\n\"UR: Send Assignment\nMacro: Pickup\""
          }
          frame True {
            n185 = case shown="True" w401 {
              tunnel: ["Macro: Analyse" ("State(s) in Front (\"\")") "Process: GO/Stop>>False" ("t")] -> w403
              frame False {
              }
              frame True {
              }
            }
          }
        }
        n186 = Bundle By Name(cluster=w392, "Assignment.GO"=w388, "Assignment.Specimen to pick"=w389) -> (w394:T2)
        n187 = call <vilib>:"Add State(s) to Queue__jki_lib_state_machine.vi"("State(s) in Front (\"\")"=w395, "State(s) in (\"\")"=w398) -> ("States Out"=w397:string)  [unwired: 13 in]
      }
      frame "Macro: Exit" {
        # "Exit Macro\n(This is called once, when the VI exits)"
        n188 = Unbundle By Name(w408) -> ("Core.Close Panel on Exit?"=w411:bool)
        n189 = call <vilib>:"Conditional State String__jki_lib_state_machine.vi"("Do State(s)?"=w411, "State"="UI: Front Panel State >> Close") -> ("State Out"=w410:string)  [unwired: 7 in]
        n190 = Bundle By Name(cluster=w408, "Core.Exit"=TRUE) -> (w407:T2)
        n191 = call <vilib>:"Add State(s) to Queue__jki_lib_state_machine.vi"("State(s) in Front (\"\")"="UI: Uninitialize\nData: Cleanup\nUI: Status>>Closing Cam connection\nCam: Uninitialize\nUI: Status>>Resetting UR\nUR: Reset\nUI: Status>>Closing UR connection\nUR: Uninitialize\nUI: Status>>See you soon" ("State(s) in Front (\"\")"), "State(s) in (\"\")"=w410, "State(s) at Back (\"\")"="Exit") -> ("States Out"=w414:string)  [unwired: 12 in]
        n192 = call <vilib>:"Add State(s) to Queue__jki_lib_state_machine.vi"("State(s) in Front (\"\")"=w414, "State(s) in (\"\")"=w417) -> ("States Out"=w416:string)  [unwired: 13 in]
      }
      frame "---------- Process ----------" {
        # "Do not put any code in this frame.\n(It is a separator no-op. You can make a copy of this frame to create a new UI frame)"
        n193 = call <vilib>:"Add State(s) to Queue__jki_lib_state_machine.vi"("State(s) in (\"\")"=w421) -> ("States Out"=w420:string)  [unwired: 14 in]
      }
      frame "Process: GO/Stop" {
        # "Do not put any code in this frame.\n(It is a separator no-op. You can make a copy of this frame to create a new UI frame)"
        n194 = case shown="\"False\", Default" w424 {
          tunnel: [FALSE ("Core.Active") TRUE ("Core.Active")] -> w423
          tunnel: ["UI: Status>>Pausing system\nUI: Cursor Set>>Idle\nUI: Buttons>>Enable" ("t") "" ("State(s) in Front (\"\")")] -> w422
          frame "False", Default {
          }
          frame "True" {
          }
        }
        n195 = Bundle By Name(cluster=w426, "Core.Active"=w423, "Assignment.GO"=w423) -> (w425:T2)
        n196 = call <vilib>:"Add State(s) to Queue__jki_lib_state_machine.vi"("State(s) in Front (\"\")"=w422, "State(s) in (\"\")"=w429) -> ("States Out"=w428:string)  [unwired: 13 in]
      }
      frame "Process: Check for Objects" {
        # "Do not put any code in this frame.\n(It is a separator no-op. You can make a copy of this frame to create a new UI frame)"
        n197 = Unbundle By Name(w436) -> ("Reshake"=w441:i32, "Sample data.Number of insects in pick-up area"=w434:i32)
        n198 = Greater Than 0?(x=w441) -> (x > 0?=w440:bool)
        n199 = Equal To 0?(x=w434) -> (x = 0?=w439:bool)
        n200 = case shown="True" w439 {
          tunnel: w441 -> [_ w450]
          tunnel: w440 -> [_ w449]
          tunnel: w438 -> [w446 _]
          tunnel: [w446 w448] -> w437
          tunnel: [0 ("Reshake") w447] -> w435
          frame False {
          }
          frame True {
            n201 = case shown="True" w449 {
              tunnel: w450 -> [_ w457]
              tunnel: [3 ("Reshake") w453] -> w447
              tunnel: ["Macro: Analyse" ("Remaining States") w454] -> w448
              frame False {
              }
              frame True {
                n202 = Equal?(x=w457, y=1) -> (x = y?=w455:bool)
                n203 = case shown="True" w455 {
                  tunnel: ["Macro: Analyse" ("Remaining States") "Macro: Exit" ("Remaining States")] -> w454
                  frame False {
                  }
                  frame True {
                  }
                }
                n204 = Decrement(x=w457) -> (x-1=w453:i32)
              }
            }
          }
        }
        n205 = Bundle By Name(cluster=w436, "Reshake"=w435) -> (w442:T2)
        n206 = call <vilib>:"Add State(s) to Queue__jki_lib_state_machine.vi"("State(s) in (\"\")"=w437) -> ("States Out"=w444:string)  [unwired: 14 in]
      }
      frame "Process: Reshape Array" {
        # "Pickup array\n(Calibrtated messurments are in real world mm);\n0. CoM X\n1. CoM Y\n2. Bounding rect. diagonal (Calibrated)\n3. Orientation"
        # "Sorted messurment array\nAll data should be reguarded as follows;\n(Calibrtated messurments are in real world mm);\n0. CoM X\n1. CoM Y\n2. Bounding rect. left (Calibrated)\n3. Bounding rect. top (Calibrated)\n4. Bounding rect. right (Calibrated)\n5. Bounding rect. buttom (Calibrated)\n6. Bounding rect. diagonal (Calibrated)\n7. Orientation\n8. Bounding rect. left\n9. Bounding rect. top\n10. Bounding rect. right\n11. Bounding rect. buttom\n12. Bounding rect. diagonal\n13. Bounding rect. center X\n14. Bounding rect. center Y\n15. Bounding rect. center X (Calibrated)\n16. Bounding rect. center Y (Calibrated)\n17. Ready for pickup"
        # "Do not put any code in this frame.\n(It is a separator no-op. You can make a copy of this frame to create a new UI frame)"
        n207 = Unbundle By Name(w466) -> ("Sample data.Raw Particle Measurements"=w464:dbl[][], "Sample data.Pixels Measurements"=w462:dbl[][])
        n208 = call "Ignore nearby.vi"("Pixel messurments"=w462, "Raw par mes."=w464) -> ("Picking array"=w461:dbl[][], "Sorted data array"=w463:dbl[][])
        n209 = call "DBL_2_STRING_ARRAY.vi"("Insect-data-array"=w461) -> ("Insect-data-array"=w460:string[][])
        "Insect-data-array" <- w460
        n210 = Bundle By Name(cluster=w466, "Sample data.Sorted Particle Measurements"=w463, "Sample data.Insect-data-array"=w460, "Sample data.Picking array"=w461) -> (w465:T2)
        n211 = call <vilib>:"Add State(s) to Queue__jki_lib_state_machine.vi"("State(s) in (\"\")"=w469) -> ("States Out"=w468:string)  [unwired: 14 in]
      }
      frame "Process: Clear Sample Data" {
        # "Do not put any code in this frame.\n(It is a separator no-op. You can make a copy of this frame to create a new UI frame)"
        n212 = Unbundle By Name(w477) -> ("Settings.Number to try and pick"=w478:i32, "Sample data.Picking array"=w472:dbl[][])
        n213 = Index Array(array=w472, index (col)=0 ("disabled index (col)")) -> (element=w473:dbl[])  [unwired: 1 in]
        n214 = Array Size(array=w473) -> (size(s)=w471:i32)
        n215 = Max & Min(x=w478, y=w471) -> (min(x,y)=w470:i32)  [unwired: 1 out]
        n216 = Bundle By Name(cluster=w477, "Sample data.Insects to pick this round"=w470, "Sample data.Insects taken from current picture"=0) -> (w476:T2)
        n217 = call <vilib>:"Add State(s) to Queue__jki_lib_state_machine.vi"("State(s) in (\"\")"=w481) -> ("States Out"=w480:string)  [unwired: 14 in]
      }
      frame "Process: Choose tool" {
        # "Do not put any code in this frame.\n(It is a separator no-op. You can make a copy of this frame to create a new UI frame)"
        n218 = Unbundle By Name(w488) -> ("Sample data.Insects to pick this round"=w483:i32, "Sample data.Picking array"=w493:dbl[][], "Settings.Tool switch size"=w495:dbl)
        n219 = for {
          N: w483 -> [w499]
          tunnel: w493 -> [w506] mode=indexing
          tunnel: w495 -> [w503]
          shift-right: [w501] -> w482
          shift-left: 0 -> [w500]
          tunnel: [w499] -> w492
          n220 = Index Array(array=w506, index=2) -> (element=w504:dbl)
          n221 = Less?(x=w504, y=w503) -> (x < y?=w502:bool)
          n222 = case shown="False" w502 {
            tunnel: [w507 w509] -> w501
            tunnel: w500 -> [w507 w508]
            frame False {
            }
            frame True {
              n223 = Increment(x=w508) -> (x+1=w509:i32)
            }
          }
        }
        n224 = Equal?(x=w492, y=w482) -> (x = y?=w491:bool)
        n225 = Greater Or Equal?(x=w482, y=3) -> (x >= y?=w489:bool)
        n226 = Compound Arithmetic op=OR(w491, w489) -> (w486:bool)
        n227 = Select(t=w482, s=w486, f=0) -> (s? t:f=w484:i32)
        n228 = Bundle By Name(cluster=w488, "Sample data.Tool1 to pick"=w484) -> (w487:T2)
        n229 = call <vilib>:"Add State(s) to Queue__jki_lib_state_machine.vi"("State(s) in (\"\")"=w498) -> ("States Out"=w497:string)  [unwired: 14 in]
      }
      frame "Process: Delay" {
        # "Do not put any code in this frame.\n(It is a separator no-op. You can make a copy of this frame to create a new UI frame)"
        n230 = Decimal String To Number(string=w511) -> (number=w510:i32)  [unwired: 2 in, 1 out]
        n231 = call "Stall Data Flow.vim"("value in"=w513, "milliseconds to wait"=w510) -> ("value out"=w512:errorcluster)  [unwired: 1 out]
        n232 = call <vilib>:"Add State(s) to Queue__jki_lib_state_machine.vi"("State(s) in (\"\")"=w516) -> ("States Out"=w515:string)  [unwired: 14 in]
      }
      frame "Process: Save Status His" {
        # "Do not put any code in this frame.\n(It is a separator no-op. You can make a copy of this frame to create a new UI frame)"
        n233 = Unbundle By Name(w522) -> ("Sample ID"=w517:string, "Core.Start Timestmap"=w530:string, "Core.Status His"=w531:string)
        n234 = call <vilib>:"Application Directory.vi"() -> ("Application Directory"=w535:path)
        n235 = Path To String(path=w535) -> (string=w519:string)
        n236 = Concatenate Strings(w519, "\\images\\phase1\\" ("string"), w517, "\\IHS_StatusHistory" ("string"), "_" ("string"), w530, ".txt" ("string")) -> (w533:string)
        n237 = String To Path(string=w533) -> (path=w523:path)
        n238 = Open/Create/Replace File(file path (use dialog)=w523, error in=w521, operation (0:open)=T7."open or create") -> (refnum out=w528:refnum<file>, error out=w527:errorcluster)  [unwired: 3 in, 1 out]
        n239 = Write to Text File(file (use dialog)=w528, text=w531, error in=w527) -> (refnum out=w525:refnum<file>, error out=w526:errorcluster)  [unwired: 1 in, 1 out]
        n240 = Close File(refnum=w525, error in=w526) -> (error out=w520:errorcluster)  [unwired: 1 out]
        n241 = call <vilib>:"Add State(s) to Queue__jki_lib_state_machine.vi"("State(s) in (\"\")"=w537) -> ("States Out"=w536:string)  [unwired: 14 in]
      }
      frame "---------- Assignment ----------" {
        # "Do not put any code in this frame.\n(It is a separator no-op. You can make a copy of this frame to create a new UI frame)"
        n242 = call <vilib>:"Add State(s) to Queue__jki_lib_state_machine.vi"("State(s) in (\"\")"=w541) -> ("States Out"=w540:string)  [unwired: 14 in]
      }
      frame "Assignment: Cam Pos" {
        # "Do not put any code in this frame.\n(It is a separator no-op. You can make a copy of this frame to create a new UI frame)"
        n243 = Unbundle By Name(w546) -> ("Core.Assignment structure"=w561:string, "Assignment.Tool"=w556:string)
        n244 = Unbundle By Name(w546) -> ("Settings.Time to Whait"=w545:dbl)
        n245 = Multiply(x=w545, y=1000.0) -> (x*y=w543:dbl)
        n246 = Number To Decimal String(number=1) -> (decimal integer string=w559:string)  [unwired: 1 in]
        n247 = Format Into String(w543) -> (resulting string=w542:string)  [unwired: 3 in, 1 out]
        n248 = Search and Replace String(input string=w561, search string="Ta", replace string=w559) -> (result string=w558:string)  [unwired: 5 in, 3 out]
        n249 = Concatenate Strings("Process: delay>>", w542) -> (w547:string)
        n250 = Search and Replace String(input string=w558, search string="To", replace string=w556) -> (result string=w555:string)  [unwired: 5 in, 3 out]
        n251 = call <vilib>:"Add State(s) to Queue__jki_lib_state_machine.vi"("State(s) in Front (\"\")"="UR: Listhen\nUR: Send Assignment" ("State(s) in Front (\"\")"), "State(s) in (\"\")"=w547) -> ("States Out"=w548:string)  [unwired: 13 in]
        n252 = Search and Replace String(input string=w555, search string="X,Y,Z,0,0,O", replace string="0,0,0,0,0,0" ("replace string (\"\")")) -> (result string=w552:string)  [unwired: 5 in, 3 out]
        n253 = Bundle By Name(cluster=w546, "Assignment.Executing Assignment"=w552) -> (w562:T2)
        n254 = call <vilib>:"Add State(s) to Queue__jki_lib_state_machine.vi"("State(s) in Front (\"\")"=w548, "State(s) in (\"\")"=w565) -> ("States Out"=w564:string)  [unwired: 13 in]
      }
      frame "Assignment: Distangle" {
        # "Selecting the apropriate distangle syckle, and forworting to the next task"
        # "Do not put any code in this frame.\n(It is a separator no-op. You can make a copy of this frame to create a new UI frame)"
        n255 = Unbundle By Name(w584) -> ("Core.Assignment structure"=w581:string, "Sample data.Number of insects in pick-up area"=w583:i32, "Settings.Last few"=w582:i32, "Assignment.Tool"=w573:string)
        n256 = First Call?() -> (First Call?: T/F=w566:bool)
        n257 = Greater?(x=w583, y=w582) -> (0:w568:bool)
        n258 = Or(x=w566, y=w568) -> (x .or. y?=w567:bool)
        n259 = Select(t=3, s=w567, f=5) -> (s? t:f=w577:i32)
        n260 = Number To Decimal String(number=w577) -> (decimal integer string=w576:string)  [unwired: 1 in]
        n261 = Search and Replace String(input string=w581, search string="Ta", replace string=w576) -> (result string=w575:string)  [unwired: 5 in, 3 out]
        n262 = Search and Replace String(input string=w575, search string="To", replace string=w573) -> (result string=w572:string)  [unwired: 5 in, 3 out]
        n263 = Search and Replace String(input string=w572, search string="X,Y,Z,0,0,O", replace string="0,0,0,0,0,0" ("replace string (\"\")")) -> (result string=w571:string)  [unwired: 5 in, 3 out]
        n264 = Bundle By Name(cluster=w584, "Assignment.Executing Assignment"=w571) -> (w585:T2)
        n265 = call <vilib>:"Add State(s) to Queue__jki_lib_state_machine.vi"("State(s) in Front (\"\")"="UR: Listhen\nUR: Send Assignment" ("State(s) in Front (\"\")"), "State(s) in (\"\")"=w589) -> ("States Out"=w588:string)  [unwired: 13 in]
      }
      frame "Assignment: Coordinates" {
        # "Do not put any code in this frame.\n(It is a separator no-op. You can make a copy of this frame to create a new UI frame)"
        n266 = Unbundle By Name(w604) -> ("Sample data.Number of insects in pick-up area"=w590:i32, "Sample data.Insects taken from current picture"=w593:i32, "Core.Assignment structure"=w595:string, "Settings.X-Zero"=w597:dbl, "Settings.Y-Zero"=w596:dbl, "Sample data.Picking array"=w605:dbl[][], "Assignment.Specimen to pick"=w594:i32)
        n267 = call "Object data correction and extraction.vi"("Cmd"=w595, "Sorted array"=w605, "Object number of interest"=w594, "y"=w596, "x"=w597) -> ("Corrected Object orientation"=w598:dbl, "Object CoM X"=w599:dbl, "Object CoM Y"=w600:dbl, "Obejct length"=w601:dbl, "Assignment Coordinates"=w602:string)
        "Length" <- w601
        "CoM Y" <- w600
        "CoM X" <- w599
        "Orientation" <- w598
        n268 = Increment(x=w593) -> (x+1=w592:i32)
        n269 = Decrement(x=w590) -> (x-1=w591:i32)
        n270 = Bundle By Name(cluster=w604, "Sample data.Number of insects in pick-up area"=w591, "Sample data.Insects taken from current picture"=w592, "Assignment.Executing Assignment"=w602, "Sample data.Object data.Object length"=w601, "Sample data.Object data.Object CoM Y"=w600, "Sample data.Object data.Object CoM X"=w599, "Sample data.Object data.Corrected Object orientation"=w598) -> (w603:T2)
        n271 = call <vilib>:"Add State(s) to Queue__jki_lib_state_machine.vi"("State(s) in (\"\")"=w608) -> ("States Out"=w607:string)  [unwired: 14 in]
      }
      frame "Assignment: Task and Tool" {
        # "Do not put any code in this frame.\n(It is a separator no-op. You can make a copy of this frame to create a new UI frame)"
        n272 = Unbundle By Name(w622) -> ("Sample data.Tool1 to pick"=w627:i32, "Sample data.Object data.Object length"=w629:dbl, "Settings.Tool switch size"=w634:dbl, "Settings.Z_Zero"=w620:dbl, "Assignment.Executing Assignment"=w631:string, "Settings.Small or XL"=w628:dbl, "Settings.Tool1-Height"=w610:dbl, "Settings.Tool2-Height"=w609:dbl)
        n273 = Greater Than 0?(x=w627) -> (x > 0?=w625:bool)
        n274 = Select(t=enum16{"Disabled", "Tool2", "Tool1"}."Tool1", s=w625, f=enum16{"Disabled", "Tool2", "Tool1"}."Tool2") -> (s? t:f=w623:enum16{"Disabled", "Tool2", "Tool1"})
        n275 = case shown="\"Tool1\", Default" w623 {
          tunnel: w634 -> [_ _ w664]
          tunnel: [w651 w658 w661] -> w611
          tunnel: [w643 w654 w662] -> w632
          tunnel: w629 -> [_ _ w663]
          tunnel: w627 -> [w647 _ _]
          tunnel: w622 -> [w650 w657 w660]
          tunnel: [w649 w657 w660] -> w621
          tunnel: w620 -> [w645 w656 w659]
          tunnel: [w646 w655 w659] -> w614
          tunnel: w610 -> [w642 _ _]
          tunnel: w609 -> [_ w652 _]
          frame "Tool1", Default {
            w644 = 1 ("f")
            n276 = Decrement(x=w647) -> (x-1=w648:i32)
            n277 = Bundle By Name(cluster=w650, "Sample data.Tool1 to pick"=w648) -> (w649:T2)
            n278 = Add(x=w642, y=w645) -> (x+y=w646:dbl)
            n279 = Format Into String(w644) -> (resulting string=w651:string)  [unwired: 3 in, 1 out]
            n280 = To Double Precision Float(number=w644) -> (double precision float=w643:dbl)
          }
          frame "Tool2" {
            w653 = 2 ("f")
            n281 = Add(x=w652, y=w656) -> (x+y=w655:dbl)
            n282 = Format Into String(w653) -> (resulting string=w658:string)  [unwired: 3 in, 1 out]
            n283 = To Double Precision Float(number=w653) -> (double precision float=w654:dbl)
          }
          frame "Disabled" {
            n284 = Greater Or Equal?(x=w663, y=w664) -> (x >= y?=w667:bool)
            n285 = Select(t=1.0 ("Tool"), s=w667, f=2.0) -> (s? t:f=w662:dbl)
            n286 = Format Into String(w662) -> (resulting string=w661:string)  [unwired: 3 in, 1 out]
          }
        }
        n287 = Divide(x=w614, y=1000.0) -> (x/y=w615:dbl)
        n288 = Format Into String(w615) -> (resulting string=w619:string)  [unwired: 3 in, 1 out]
        n289 = Search and Replace String(input string=w631, search string="To", replace string=w611) -> (result string=w630:string)  [unwired: 5 in, 3 out]
        n290 = Search and Replace String(input string=w619, search string=",", replace string="." ("replace string (\"\")")) -> (result string=w616:string)  [unwired: 5 in, 3 out]
        n291 = Search and Replace String(input string=w630, search string="Z", replace string=w616) -> (result string=w635:string)  [unwired: 5 in, 3 out]
        n292 = call "Task from tool.vi"("Too large"=w628, "Object lengh"=w629, "Tool"=w632, "Assignment - Task"=w635) -> ("Task to String"=w612:string, "Assignment"=w637:string)  [unwired: 6 in]
        n293 = Bundle By Name(cluster=w621, "Assignment.Executing Assignment"=w637, "Assignment.Task"=w612, "Assignment.Tool"=w611) -> (w638:T2)
        n294 = call <vilib>:"Add State(s) to Queue__jki_lib_state_machine.vi"("State(s) in (\"\")"=w641) -> ("States Out"=w640:string)  [unwired: 14 in]
      }
      frame "---------- IA ----------" {
        # "Do not put any code in this frame.\n(It is a separator no-op. You can make a copy of this frame to create a new UI frame)"
        n295 = call <vilib>:"Add State(s) to Queue__jki_lib_state_machine.vi"("State(s) in (\"\")"=w671) -> ("States Out"=w670:string)  [unwired: 14 in]
      }
      frame "IA: Analyse Image" {
        # "Do not put any code in this frame.\n(It is a separator no-op. You can make a copy of this frame to create a new UI frame)"
        n296 = Unbundle By Name(w689) -> ("Images.Image"=w694:T1, "Core.Close Panel on Exit?"=w680:bool, "Settings.Ignore small"=w672:dbl)
        n297 = Bundle By Name(cluster=T8 {"Measurement Parameter"=18, "Range Lower Value"=0.0, "Range Upper Value"=0.5, "Range"=FALSE, "Measurement Type"=TRUE} ("Selection Value"), "Range Upper Value"=w672) -> (w674:T8)
        n298 = case shown="True" w680 {
          tunnel: [path "C:/Projects/BioDiscover/src/LabVIEW/IHS/assets/Grid calibration.png" w697] -> w681
          frame False {
          }
          frame True {
            n299 = call <vilib>:"Application Directory.vi"() -> ("Application Directory"=w701:path)
            n300 = Path To String(path=w701) -> (string=w700:string)
            n301 = Concatenate Strings(w700, "\\data\\Grid calibration.png") -> (w698:string)
            n302 = String To Path(string=w698) -> (path=w697:path)
          }
        }
        n303 = Build Array(w674) -> (w673:T10)
        n304 = call "Vision Assistant3"("Image In"=w694, "Selection Values (Particle Filter 2 Remove small)"=w673, "File Path (Image Calibration 1)"=w681, "error in"=w693) -> ("Image Out"=w688:T1, "Number of Particles (Particle Analysis 1)"=w685:i32, "Particle Measurements (Real-World) (Particle Analysis 1)"=w687:dbl[][], "Match Score (Color Matching 1)"=w690:i32[], "Particle Measurements (Pixels) (Particle Analysis 1)"=w686:dbl[][], "error out"=w692:errorcluster)  [unwired: 18 in]
        "Vision A. Image" <- w688
        "Number of objects" <- w685
        n305 = call "Black_image_detection.vi"("Match score"=w690) -> ("No Error"=w691:bool)  [unwired: 1 in]
        n306 = feedback #2(0.0) -> (w677:dbl)
        n307 = case shown="False" w691 {
          tunnel: w689 -> [w708 w726]
          tunnel: w688 -> [_ w725]
          tunnel: w687 -> [_ w724]
          tunnel: w686 -> [_ w723]
          tunnel: w685 -> [_ w722]
          tunnel: [w708 w720] -> w684
          tunnel: w683 -> [w703 w721]
          tunnel: [w709 w721] -> w682
          tunnel: [w704 0.0] -> w679
          tunnel: w677 -> [w705 _]
          tunnel: [w702 "" ("State(s) in Front (\"\")")] -> w676
          frame False {
            n308 = Greater Or Equal?(x=w705, y=3.0) -> (x >= y?=w706:bool)
            n309 = case shown="True" w706 {
              tunnel: [w711 "Process: GO/Stop>>False" ("Remaining States")] -> w709
              tunnel: w705 -> [w713 _]
              tunnel: [w712 0.0] -> w704
              tunnel: w703 -> [w711 _]
              tunnel: ["Cam: Grap Image\nIA: Analyse Image" ("State(s) in Front (\"\")") "" ("State(s) in Front (\"\")")] -> w702
              frame False {
                n310 = Increment(x=w713) -> (x+1=w712:dbl)
              }
              frame True {
                n311 = One Button Dialog(message="Black Image Error") -> ()  [unwired: 1 in, 1 out]
              }
            }
          }
          frame True {
            n312 = Bundle By Name(cluster=w726, "Images.Vision A. Image"=w725, "Sample data.Raw Particle Measurements"=w724, "Sample data.Pixels Measurements"=w723, "Sample data.Number of insects in pick-up area"=w722) -> (w720:T2)
          }
        }
        n313 = feedback-in #2(w679) -> ()
        n314 = call <vilib>:"Add State(s) to Queue__jki_lib_state_machine.vi"("State(s) in Front (\"\")"=w676, "State(s) in (\"\")"=w682) -> ("States Out"=w695:string)  [unwired: 13 in]
      }
      frame "IA: Draw borders" {
        # "Do not put any code in this frame.\n(It is a separator no-op. You can make a copy of this frame to create a new UI frame)"
        n315 = Unbundle By Name(w733) -> ("Images.Image"=w736:T1, "Sample data.Sorted Particle Measurements"=w730:dbl[][], "Sample data.Number of insects in pick-up area"=w729:i32)
        n316 = Greater?(x=w729, y=0) -> (0:w727:bool)
        n317 = case shown="True" w727 {
          tunnel: w736 -> [w740 w741]
          tunnel: w730 -> [_ w751]
          tunnel: w735 -> [w739 w742]
          tunnel: [w739 w750] -> w734
          tunnel: [w740 w743] -> w731
          frame False {
          }
          frame True {
            w744 = T11 4 items=["Grayscale (U8)", "Grayscale (I16)", "Grayscale (SGL)", "Complex (CSG)", "RGB (U32)", "HSL (U32)", "RGB (U64)", "Grayscale (U16)"] ("Image Type")
            n318 = for {
              tunnel: w742 -> [w771]
              shift-right: [w769] -> w749
              shift-left: w741 -> [w772]
              tunnel: w751 -> [w765] mode=indexing
              tunnel: [w770] -> w748
              w768 = u32 0 items=["Frame", "Fill"] ("Drawing Mode (Frame)")
              n319 = Index Array(array=w765, index #1=8 ("index"), index #5=17 ("index")) -> (element #1=w755:dbl, element #2=w754:dbl, element #3=w753:dbl, element #4=w752:dbl, element #5=w756:dbl)  [unwired: 3 in]
              n320 = To Long Integer(number=w756) -> (32bit integer=w763:i32)
              n321 = To Long Integer(number=w753) -> (32bit integer=w760:i32)
              n322 = To Long Integer(number=w754) -> (32bit integer=w761:i32)
              n323 = To Long Integer(number=w755) -> (32bit integer=w762:i32)
              n324 = To Long Integer(number=w752) -> (32bit integer=w759:i32)
              n325 = case shown="1" w763 {
                tunnel: [u32 16711680 ("Text Color (black)") u32 6618880 ("Text Color (black)")] -> w764
                frame 0, Default {
                }
                frame 1 {
                }
              }
              n326 = Bundle By Name(cluster=T9 {"Left"=0, "Top"=0, "Right"=0, "Bottom"=0} ("Bounding Rectangle"), "Left"=w762, "Top"=w761, "Right"=w760, "Bottom"=w759) -> (w766:T9)
              n327 = call "IMAQ Overlay Oval"("Color"=w764, "error in (no error)"=w771, "Drawing Mode (Frame)"=w768, "Bounding Rectangle"=w766, "Image"=w772) -> ("error out"=w770:errorcluster, "Image Out"=w769:T1)  [unwired: 5 in]
            }
            n328 = call "IMAQ Create"("Image Name"="Image borders", "Image Type"=w744, "error in (no error)"=w748) -> ("New Image"=w746:T1, "error out"=w747:errorcluster)  [unwired: 2 in]
            n329 = call "IMAQ Merge Overlay"("error in (no error)"=w747, "Image Dst"=w746, "Image Src"=w749) -> ("error out"=w750:errorcluster, "Image Dst Out"=w743:T1)  [unwired: 7 in]
            n330 = local write "Camera feed"(w743) -> ()
          }
        }
        n331 = Bundle By Name(cluster=w733, "Images.Boarder Image"=w731) -> (w732:T2)
        n332 = call <vilib>:"Add State(s) to Queue__jki_lib_state_machine.vi"("State(s) in (\"\")"=w738) -> ("States Out"=w737:string)  [unwired: 14 in]
      }
      frame "---------- Cam ----------" {
        # "Template Separator\n(You can make a copy of, or modify, this frame)"
        n333 = call <vilib>:"Add State(s) to Queue__jki_lib_state_machine.vi"("State(s) in (\"\")"=w778) -> ("States Out"=w777:string)  [unwired: 14 in]
      }
      frame "Cam: Initialize" {
        w791 = T11 4 items=["Grayscale (U8)", "Grayscale (I16)", "Grayscale (SGL)", "Complex (CSG)", "RGB (U32)", "HSL (U32)", "RGB (U64)", "Grayscale (U16)"] ("Image Type")
        # "Camera initialization"
        # "Your code here.\n(You can make a copy of, or modify, this frame)"
        n334 = call <vilib>:"IMAQdx Enumerate Cameras.vi"("error in"=w787) -> ("error out"=w782:errorcluster, "Camera Information Array"=w784:T12)  [unwired: 9 in]
        n335 = while {
          tunnel: w784 -> [w809]
          tunnel: "Blackfly" ("regular expression") -> [w802]
          tunnel: w782 -> [w798]
          tunnel: [w797] -> w779
          tunnel: [w796] -> w781
          tunnel: [w795] -> w780
          i -> [w807]
          stop <- w806 stop-if-true
          n336 = Array Size(array=w809) -> (size(s)=w808:i32)
          n337 = Greater?(x=w807, y=w808) -> (0:w805:bool)
          n338 = Index Array(array=w809, index=w807) -> (element=w801:T13)
          n339 = Unbundle By Name(w801) -> ("ModelName"=w803:string, "InterfaceName"=w799:string)
          n340 = Match True/False String(2:"" ("false string"), 3:w802, 4:w803) -> (0:w800:bool)  [unwired: 1 out]
          n341 = case shown="True" w800 {
            tunnel: w799 -> [_ w818]
            tunnel: w798 -> [w811 w817]
            tunnel: [w811 w815] -> w797
            tunnel: [T3 refnum ("Session Out") w814] -> w796
            tunnel: [FALSE TRUE ("Cam.Connected")] -> w795
            frame False {
            }
            frame True {
              n342 = call <vilib>:"IMAQdx Open Camera.vi"("error in"=w817, "Session In"=w818) -> ("error out"=w816:errorcluster, "Session Out"=w819:T3)  [unwired: 8 in]
              n343 = call <vilib>:"IMAQdx Configure Grab.vi"("error in"=w816, "Session In"=w819) -> ("error out"=w815:errorcluster, "Session Out"=w814:T3)  [unwired: 8 in]
            }
          }
          n344 = Or(x=w795, y=w805) -> (x .or. y?=w806:bool)
        }
        "Cam Connection" <- w780
        n345 = call "IMAQ Create"("Image Name"="Picture", "Image Type"=w791, "error in (no error)"=w787) -> ("New Image"=w788:T1, "error out"=w786:errorcluster)  [unwired: 2 in]
        n346 = Bundle By Name(cluster=w790, "Cam.Cam"=w781, "Images.Image"=w788, "Cam.Connected"=w780) -> (w789:T2)
        n347 = Merge Errors(w786, w779) -> (w785:errorcluster)
        n348 = call <vilib>:"Add State(s) to Queue__jki_lib_state_machine.vi"("State(s) in (\"\")"=w794) -> ("States Out"=w793:string)  [unwired: 14 in]
      }
      frame "Cam: Grap Image" {
        # "Template Separator\n(You can make a copy of, or modify, this frame)"
        n349 = Unbundle By Name(w825) -> ("Cam.Save pictures"=w822:bool, "Cam.Cam"=w823:T3, "Images.Image"=w824:T1, "Cam.Connected"=w820:bool)
        n350 = case shown="True" w820 {
          tunnel: w828 -> [w831 w847]
          tunnel: [w831 w846] -> w827
          tunnel: [w833 w845] -> w826
          tunnel: w825 -> [w833 w842]
          tunnel: w824 -> [_ w841]
          tunnel: w823 -> [_ w840]
          tunnel: w822 -> [_ w835]
          tunnel: ["" ("States Out") w834] -> w821
          frame False {
          }
          frame True {
            # "Get picture \nfrom camera"
            # "Rotate image"
            n351 = call <vilib>:"IMAQdx Grab2.vi"("error in"=w847, "Image In"=w841, "Session In"=w840) -> ("error out"=w846:errorcluster, "Image Out"=w850:T1, "Session Out"=w844:T3)  [unwired: 5 in, 1 out]
            n352 = call-poly <vilib>:"Select State(s)__jki_lib_state_machine.vi"("State(s) if True (\"\")"="Cam: Save Image" ("State(s) if True (\"\")"), "Select"=w835) -> ("States Out"=w834:string)  [unwired: 13 in]
            n353 = call "IMAQ Rotate"("Maintain Size"=TRUE, "Angle (degrees)"=sgl 270.0, "Image Src"=w850) -> ("Image Dst Out"=w843:T1)  [unwired: 7 in, 1 out]
            "Camera feed" <- w843
            n354 = Format Date/Time String(time format string (%c)="%Y-%m-%d_%H;%M;%S%3u", UTC format=FALSE) -> (date/time string=w837:string)  [unwired: 1 in]
            n355 = Bundle By Name(cluster=w842, "Cam.Cam"=w844, "Images.Image"=w843, "Images.Image Timestamp"=w837) -> (w845:T2)
          }
        }
        n356 = call <vilib>:"Add State(s) to Queue__jki_lib_state_machine.vi"("State(s) in Front (\"\")"=w821, "State(s) in (\"\")"=w830) -> ("States Out"=w829:string)  [unwired: 13 in]
      }
      frame "Cam: Select test image" {
        w862 = T11 4 items=["Grayscale (U8)", "Grayscale (I16)", "Grayscale (SGL)", "Complex (CSG)", "RGB (U32)", "HSL (U32)", "RGB (U64)", "Grayscale (U16)"] ("Image Type")
        # "Template Separator\n(You can make a copy of, or modify, this frame)"
        n357 = call <vilib>:"Application Directory.vi"() -> ("Application Directory"=w869:path)
        n358 = Path To String(path=w869) -> (string=w868:string)
        n359 = Concatenate Strings(w868, "\\" ("string")) -> (w867:string)
        n360 = String To Path(string=w867) -> (path=w865:path)
        n361 = call "File Dialog"("start path"=w865, "error in"=w855, "pattern (all files)"="*.png*") -> ("selected path"=w864:path, "error out"=w860:errorcluster)  [unwired: 9 in, 2 out]
        n362 = call "IMAQ Create"("Image Name"="Test", "Image Type"=w862, "error in (no error)"=w860) -> ("New Image"=w861:T1, "error out"=w859:errorcluster)  [unwired: 2 in]
        n363 = Format Date/Time String(time format string (%c)="%Y-%m-%d_%H;%M;%S%3u", UTC format=FALSE) -> (date/time string=w858:string)  [unwired: 1 in]
        n364 = call "IMAQ ReadFile 2"("File Path"=w864, "error in (no error)"=w859, "Image"=w861) -> ("error out"=w854:errorcluster, "Image Out"=w851:T1)  [unwired: 4 in, 3 out]
        n365 = local write "Camera feed"(w851) -> ()
        n366 = Concatenate Strings("TEST_" ("string"), w858) -> (w856:string)
        n367 = Bundle By Name(cluster=w853, "Images.Image"=w851, "Images.Image Timestamp"=w856) -> (w852:T2)
        n368 = call <vilib>:"Add State(s) to Queue__jki_lib_state_machine.vi"("State(s) in (\"\")"=w874) -> ("States Out"=w873:string)  [unwired: 14 in]
      }
      frame "Cam: Save Image" {
        # "Template Separator\n(You can make a copy of, or modify, this frame)"
        n369 = Unbundle By Name(w882) -> ("Images.Image"=w876:T1, "Sample ID"=w881:string, "Images.Image Timestamp"=w875:string)
        n370 = call <vilib>:"Application Directory.vi"() -> ("Application Directory"=w883:path)
        n371 = Search and Replace String(input string=w875, search string=":", replace string="_" ("replace string (\"\")")) -> (result string=w885:string)  [unwired: 5 in, 3 out]
        n372 = Path To String(path=w883) -> (string=w893:string)
        n373 = Search and Replace String(input string=w885, search string=":", replace string="_" ("replace string (\"\")")) -> (result string=w884:string)  [unwired: 5 in, 3 out]
        n374 = Concatenate Strings(w893, "\\images\\phase1\\" ("string"), w881) -> (w898:string)
        n375 = String To Path(string=w898) -> (path=w897:path)
        n376 = call <vilib>:"Check if File or Folder Exists.vi"("error in (no error)"=w880, "path"=w897) -> ("error out"=w879:errorcluster, "file or folder exists?"=w896:bool, "dup path"=w895:path)  [unwired: 7 in]
        n377 = case shown="True" w896 {
          tunnel: w895 -> [w907 w909]
          tunnel: [w906 w909] -> w899
          tunnel: w879 -> [w905 w908]
          tunnel: [w904 w908] -> w878
          frame False {
            n378 = Create Folder(path (use dialog)=w907, error in=w905) -> (created path=w906:path, error out=w904:errorcluster)  [unwired: 1 in, 1 out]
          }
          frame True {
          }
        }
        n379 = Path To String(path=w899) -> (string=w891:string)
        n380 = Concatenate Strings(w891, "\\" ("string"), w884, ".png" ("string")) -> (w901:string)
        n381 = String To Path(string=w901) -> (path=w900:path)
        n382 = call-poly "IMAQ Write File 2"("error in (no error)"=w878, "File Path"=w900, "Image"=w876) -> ("error out"=w877:errorcluster)  [unwired: 7 in, 1 out]
        n383 = call <vilib>:"Add State(s) to Queue__jki_lib_state_machine.vi"("State(s) in (\"\")"=w903) -> ("States Out"=w902:string)  [unwired: 14 in]
      }
      frame "Cam: Uninitialize" {
        # "Your code here.\n(You can make a copy of, or modify, this frame)"
        n384 = Unbundle By Name(w911) -> ("Cam.Cam"=w914:T3, "Images.Image"=w915:T1, "Cam.Connected"=w916:bool)
        n385 = case shown="True" w916 {
          tunnel: w915 -> [_ w931]
          tunnel: w914 -> [_ w930]
          tunnel: w912 -> [w919 w929]
          tunnel: [w919 w926] -> w913
          tunnel: w911 -> [w920 w925]
          tunnel: [w920 w923] -> w910
          frame False {
          }
          frame True {
            w922 = FALSE ("Cam.Connected")
            n386 = call "Imaq Dispose"("All Images? (No)"=TRUE, "Image"=w931, "error in (no error)"=w929) -> ("error out"=w928:errorcluster)  [unwired: 3 in]
            n387 = call <vilib>:"IMAQdx Close Camera.vi"("error in"=w929, "Session In"=w930) -> ("error out"=w927:errorcluster)  [unwired: 9 in]
            n388 = Merge Errors(w928, w927) -> (w926:errorcluster)
            n389 = Bundle By Name(cluster=w925, "Cam.Cam"=T3 refnum, "Images.Image"=T1 refnum ("Cam.Image"), "Cam.Connected"=w922) -> (w923:T2)
            n390 = local write "Cam Connection"(w922) -> ()
          }
        }
        n391 = call <vilib>:"Add State(s) to Queue__jki_lib_state_machine.vi"("State(s) in (\"\")"=w918) -> ("States Out"=w917:string)  [unwired: 14 in]
      }
      frame "---------- UR ----------" {
        # "Template Separator\n(You can make a copy of, or modify, this frame)"
        n392 = call <vilib>:"Add State(s) to Queue__jki_lib_state_machine.vi"("State(s) in (\"\")"=w936) -> ("States Out"=w935:string)  [unwired: 14 in]
      }
      frame "UR: Initialize" {
        # "Template Separator\n(You can make a copy of, or modify, this frame)"
        n393 = Unbundle By Name(w942) -> ("UR.PC_IP"=w946:string, "UR.UR_IP"=w944:string, "UR.Remote port"=w943:u16)
        n394 = String To IP(1:w946) -> (0:w945:u32)
        n395 = call <vilib>:"TCP Listen.vi"("net address"=w945, "error in (no error)"=w947, "timeout ms (wait forever: -1)"=10000, "port"=w943, "service name"=w944) -> ("error out"=w940:errorcluster, "connection ID"=w941:refnum<k5>)  [unwired: 2 in, 3 out]
        n396 = case shown="Error .." w940 {
          tunnel: w942 -> [w955 w958]
          tunnel: w941 -> [w954 _]
          tunnel: [w953 w957] -> w939
          tunnel: ["Data: Save Settings" ("State(s) in Front (\"\")") "" ("State(s) in Front (\"\")")] -> w938
          tunnel: [w951 w956] -> w937
          frame No Error {
            w951 = TRUE ("UR.Connected")
            n397 = Bundle By Name(cluster=w955, "UR.connection ID"=w954, "UR.Connected"=w951) -> (w953:T2)
          }
          frame Error {
            w956 = FALSE ("UR.Connected")
            n398 = Bundle By Name(cluster=w958, "UR.Connected"=w956) -> (w957:T2)
          }
        }
        "UR Connection" <- w937
        n399 = call <vilib>:"Add State(s) to Queue__jki_lib_state_machine.vi"("State(s) in Front (\"\")"=w938, "State(s) in (\"\")"=w950) -> ("States Out"=w949:string)  [unwired: 13 in]
      }
      frame "UR: Listhen" {
        # "Template Separator\n(You can make a copy of, or modify, this frame)"
        n400 = Unbundle By Name(w963) -> ("UR.connection ID"=w964:refnum<k5>, "UR.Sim UR signal"=w961:bool, "UR.Connected"=w960:bool)
        n401 = case shown="True" w960 {
          tunnel: w966 -> [w969 w983]
          tunnel: [w969 w982] -> w965
          tunnel: w964 -> [_ w981]
          tunnel: w963 -> [w972 w973]
          tunnel: [w971 w977] -> w962
          tunnel: w961 -> [w970 w980]
          frame False {
            n402 = Bundle By Name(cluster=w972, "UR.UR Ready"=w970) -> (w971:T2)
          }
          frame True {
            n403 = while {
              tunnel: w983 -> [w1007]
              tunnel: [w1006] -> w982
              tunnel: w981 -> [w1005]
              tunnel: [w996] -> w979
              tunnel: w980 -> [w995]
              i -> [w1002]
              stop <- w998 stop-if-true
              n404 = Wait (ms)(milliseconds to wait=u32 250) -> ()  [unwired: 1 out]
              n405 = Greater?(x=w1002, y=20) -> (0:w999:bool)
              n406 = call "Robot_listen.vi"("error in (no error)"=w1007, "connection ID IN"=w1005) -> ("error IO"=w1006:errorcluster, "robotmessage"=w1004:string)  [unwired: 7 in, 1 out]
              "Robotmessage" <- w1004
              n407 = Equal?(x="Done", y=w1004) -> (x = y?=w997:bool)
              n408 = Or(x=w995, y=w997) -> (x .or. y?=w996:bool)
              n409 = Or(x=w996, y=w999) -> (x .or. y?=w998:bool)
            }
            "UR-Ready" <- w979
            n410 = Unbundle By Name(w973) -> ("UR.Ready fail"=w978:dbl)
            n411 = case shown="True" w979 {
              tunnel: w978 -> [w988 _]
              tunnel: [w987 0.0 ("UR.Ready fail")] -> w976
              tunnel: [FALSE w993] -> w975
              tunnel: [w984 w993] -> w974
              frame False {
                n412 = Greater Or Equal?(x=w988, y=5.0) -> (x >= y?=w986:bool)
                n413 = case shown="True" w986 {
                  tunnel: [TRUE FALSE] -> w984
                  frame False {
                  }
                  frame True {
                    n414 = One Button Dialog(message="UR signal failed 5 times. \nConnection terminated.") -> ()  [unwired: 1 in, 1 out]
                  }
                }
                n415 = Increment(x=w988) -> (x+1=w987:dbl)
              }
              frame True {
                w993 = TRUE
              }
            }
            n416 = Bundle By Name(cluster=w973, "UR.UR Ready"=w975, "UR.Ready fail"=w976, "UR.Connected"=w974) -> (w977:T2)
          }
        }
        n417 = call <vilib>:"Add State(s) to Queue__jki_lib_state_machine.vi"("State(s) in (\"\")"=w968) -> ("States Out"=w967:string)  [unwired: 14 in]
      }
      frame "UR: Send Assignment" {
        # "Template Separator\n(You can make a copy of, or modify, this frame)"
        n418 = Unbundle By Name(w1011) -> ("UR.connection ID"=w1014:refnum<k5>, "Assignment.Executing Assignment"=w1015:string, "UR.UR Ready"=w1013:bool, "UR.Connected"=w1008:bool, "UR.Sim UR signal"=w1009:bool)
        n419 = case shown="True" w1008 {
          tunnel: w1017 -> [w1025 w1041]
          tunnel: [w1025 w1040] -> w1016
          tunnel: w1015 -> [w1023 w1039]
          tunnel: w1014 -> [_ w1038]
          tunnel: w1013 -> [_ w1037]
          tunnel: [w1022 w1036] -> w1012
          tunnel: w1011 -> [w1021 w1035]
          tunnel: [w1020 w1034] -> w1010
          tunnel: w1009 -> [w1024 _]
          frame False {
            n420 = case shown="False" w1024 {
              tunnel: w1023 -> [_ w1031]
              tunnel: ["" w1032] -> w1022
              tunnel: w1021 -> [w1026 w1030]
              tunnel: [w1026 w1029] -> w1020
              frame False {
              }
              frame True {
                n421 = local write "Executing Assignment"(w1031) -> ()
                n422 = Bundle By Name(cluster=w1030, "Assignment.GO"=FALSE) -> (w1029:T2)
                n423 = Concatenate Strings("UI: Status>>SIM CMD;" ("State(s) in Front (\"\")"), w1031) -> (w1032:string)
              }
            }
          }
          frame True {
            n424 = case shown="True" w1037 {
              tunnel: w1041 -> [w1044 w1054]
              tunnel: [w1044 w1053] -> w1040
              tunnel: w1039 -> [_ w1046]
              tunnel: w1038 -> [_ w1052]
              tunnel: ["UR: Listhen\nUR: Send Assignment" ("State(s) in Front (\"\")") w1047] -> w1036
              tunnel: w1035 -> [w1042 w1050]
              tunnel: [w1042 w1049] -> w1034
              frame False {
              }
              frame True {
                w1045 = FALSE ("UR Ready")
                n425 = call "robot_comSUBVI.vi"("error in (no error)"=w1054, "message"=w1046, "ConnectionID In"=w1052) -> ("error IO"=w1053:errorcluster, "robotmessage"=w1051:string)  [unwired: 6 in, 1 out]
                n426 = local write "Robotmessage"(w1051) -> ()
                n427 = local write "UR-Ready"(w1045) -> ()
                n428 = Bundle By Name(cluster=w1050, "Assignment.GO"=w1045, "UR.UR Ready"=w1045) -> (w1049:T2)
                n429 = Concatenate Strings("UI: Status>>CMD;" ("State(s) in Front (\"\")"), w1046) -> (w1047:string)
                "Executing Assignment" <- w1046
              }
            }
          }
        }
        n430 = call <vilib>:"Add State(s) to Queue__jki_lib_state_machine.vi"("State(s) in Front (\"\")"=w1012, "State(s) in (\"\")"=w1019) -> ("States Out"=w1018:string)  [unwired: 13 in]
      }
      frame "UR: Reset" {
        # "Template Separator\n(You can make a copy of, or modify, this frame)"
        n431 = Unbundle By Name(w1056) -> ("UR.Connected"=w1055:bool)
        n432 = case shown="True" w1055 {
          tunnel: w1056 -> [w1063 w1067]
          tunnel: [w1063 w1066] -> w1058
          tunnel: ["" ("State(s) in Front (\"\")") "UR: Send Assignment" ("State(s) in Front (\"\")")] -> w1057
          frame False {
          }
          frame True {
            n433 = Bundle By Name(cluster=w1067, "Assignment.Executing Assignment"="(55,0,0,0,0,0,0,0)") -> (w1066:T2)
          }
        }
        n434 = call <vilib>:"Add State(s) to Queue__jki_lib_state_machine.vi"("State(s) in Front (\"\")"=w1057, "State(s) in (\"\")"=w1061) -> ("States Out"=w1060:string)  [unwired: 13 in]
      }
      frame "UR: Uninitialize" {
        # "Template Separator\n(You can make a copy of, or modify, this frame)"
        n435 = Unbundle By Name(w1070) -> ("UR.connection ID"=w1068:refnum<k5>, "UR.Connected"=w1069:bool)
        n436 = case shown="True" w1069 {
          tunnel: w1070 -> [w1077 w1079]
          tunnel: [w1077 w1084] -> w1073
          tunnel: w1072 -> [w1076 w1083]
          tunnel: [w1076 w1082] -> w1071
          tunnel: w1068 -> [_ w1080]
          frame False {
          }
          frame True {
            w1078 = FALSE ("UR.Connected")
            n437 = TCP Close Connection(connection ID=w1080, error in (no error)=w1083) -> (connection ID out=w1081:refnum<k5>, error out=w1082:errorcluster)  [unwired: 1 in]
            n438 = Bundle By Name(cluster=w1079, "UR.connection ID"=w1081, "Cam.Connected"=w1078) -> (w1084:T2)
            n439 = local write "UR Connection"(w1078) -> ()
          }
        }
        n440 = call <vilib>:"Add State(s) to Queue__jki_lib_state_machine.vi"("State(s) in (\"\")"=w1075) -> ("States Out"=w1074:string)  [unwired: 14 in]
      }
    }
  }
